vi "Waveform 64-128 channels LP pt by pt Prefilter 2.vi"(6 "order":i32=2, 8 "fl":dbl, 10 "fs":dbl, 11 "Array in":waveform(dbl)[](array[waveform])) -> (3 "Array out":waveform(dbl)[](array[waveform]))   [LabVIEW 2013]
uses:
  <vilib>/Analysis/3filter.llb/Filter Passband Type.ctl
  <vilib>/ptbypt/NI_PtbyPt.lvlib
  <vilib>/Analysis/NI_AALBase.lvlib
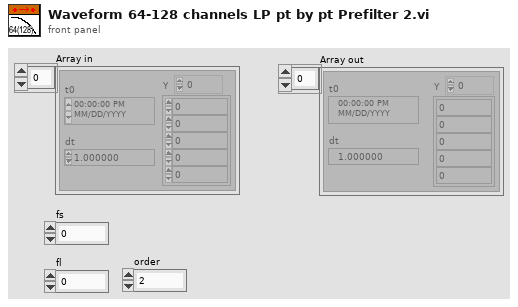
[diagram p1: front panel]
types:
  T1 = typedef "NI_AALBase.lvlib/Filter Passband Type.ctl" = enum32{"Lowpass", "Highpass", "Bandpass", "Bandstop"}
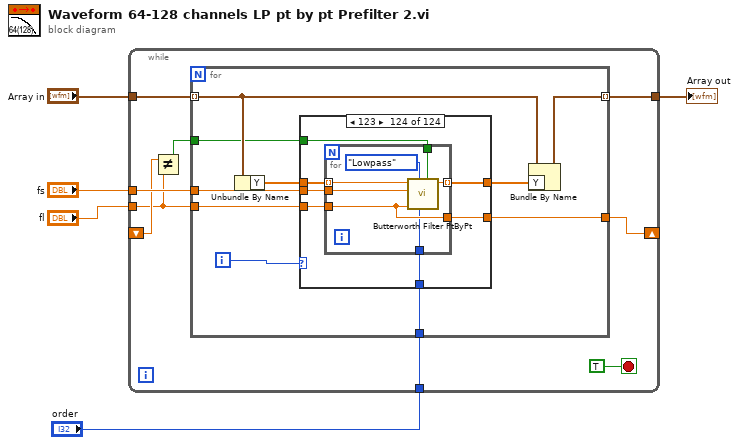
[diagram p0: block diagram]
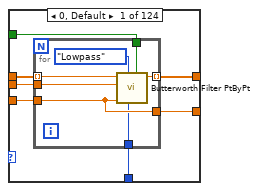
[diagram p2: hidden frame]
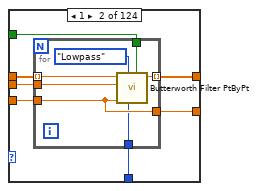
[diagram p3: hidden frame]
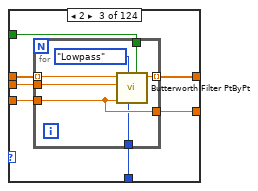
[diagram p4: hidden frame]
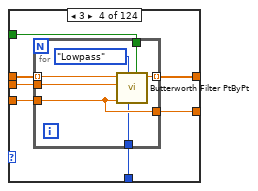
[diagram p5: hidden frame]
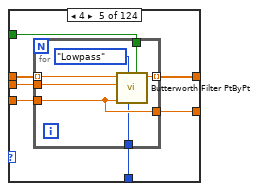
[diagram p6: hidden frame]
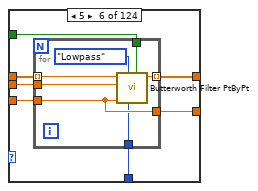
[diagram p7: hidden frame]
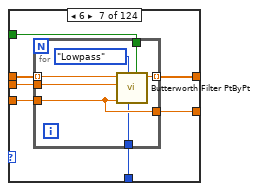
[diagram p8: hidden frame]
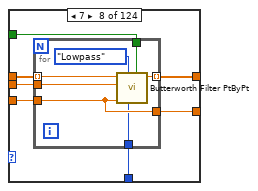
[diagram p9: hidden frame]
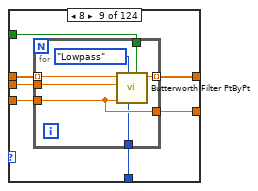
[diagram p10: hidden frame]
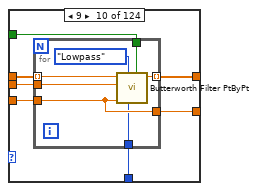
[diagram p11: hidden frame]
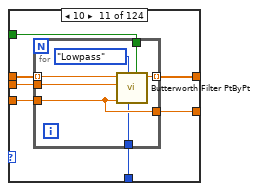
[diagram p12: hidden frame]
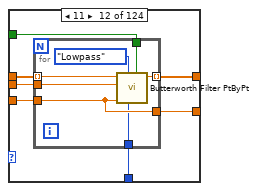
[diagram p13: hidden frame]
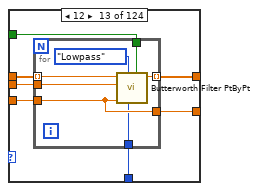
[diagram p14: hidden frame]
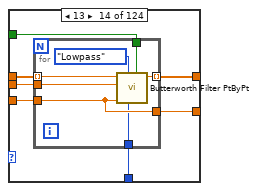
[diagram p15: hidden frame]
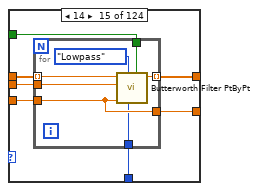
[diagram p16: hidden frame]
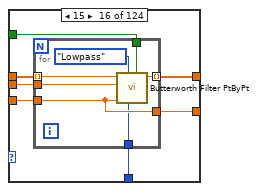
[diagram p17: hidden frame]
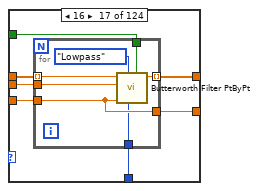
[diagram p18: hidden frame]
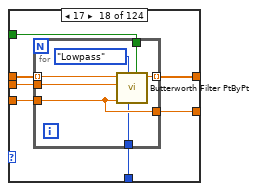
[diagram p19: hidden frame]
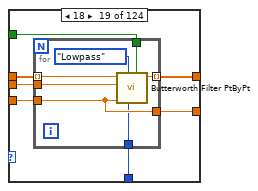
[diagram p20: hidden frame]
diagram:
  n1 = while {
    tunnel: "Array in" -> [w14]
    tunnel: [w13] -> w4
    tunnel: "fs" -> [w10]
    tunnel: "fl" -> [w7]
    shift-right: [w11] -> _
    shift-left: _ -> [w9]
    tunnel: "order" -> [w8]
    stop <- TRUE stop-if-true
    n2 = Not Equal?(x=w9, y=w7) -> (x != y?=w6:bool)
    n3 = for {
      tunnel: w14 -> [w22] mode=indexing
      tunnel: w10 -> [w24]
      tunnel: [w23] -> w13 mode=indexing
      tunnel: w7 -> [w21]
      tunnel: [w20] -> w11
      tunnel: w6 -> [w19]
      tunnel: w8 -> [w18]
      i -> [w15]
      n4 = Unbundle By Name(w22) -> ("Y"=w16:dbl[])
      n5 = case shown="123" w15 {
        tunnel: w24 -> [w31 w45 w59 w73 w87 w101 w115 w129 w143 w157 w171 w185 w199 w213 w227 w241 w255 w269 w283 w297 w311 w325 w339 w353 w367 w381 w395 w409 w423 w437 w451 w465 w479 w493 w507 w521 w535 w549 w563 w577 w591 w605 w619 w633 w647 w661 w675 w689 w703 w717 w731 w745 w759 w773 w787 w801 w815 w829 w843 w857 w871 w885 w899 w913 w927 w941 w955 w969 w983 w997 w1011 w1025 w1039 w1053 w1067 w1081 w1095 w1109 w1123 w1137 w1151 w1165 w1179 w1193 w1207 w1221 w1235 w1249 w1263 w1277 w1291 w1305 w1319 w1333 w1347 w1361 w1375 w1389 w1403 w1417 w1431 w1445 w1459 w1473 w1487 w1501 w1515 w1529 w1543 w1557 w1571 w1585 w1599 w1613 w1627 w1641 w1655 w1669 w1683 w1697 w1711 w1725 w1739 w1753]
        tunnel: w21 -> [w30 w44 w58 w72 w86 w100 w114 w128 w142 w156 w170 w184 w198 w212 w226 w240 w254 w268 w282 w296 w310 w324 w338 w352 w366 w380 w394 w408 w422 w436 w450 w464 w478 w492 w506 w520 w534 w548 w562 w576 w590 w604 w618 w632 w646 w660 w674 w688 w702 w716 w730 w744 w758 w772 w786 w800 w814 w828 w842 w856 w870 w884 w898 w912 w926 w940 w954 w968 w982 w996 w1010 w1024 w1038 w1052 w1066 w1080 w1094 w1108 w1122 w1136 w1150 w1164 w1178 w1192 w1206 w1220 w1234 w1248 w1262 w1276 w1290 w1304 w1318 w1332 w1346 w1360 w1374 w1388 w1402 w1416 w1430 w1444 w1458 w1472 w1486 w1500 w1514 w1528 w1542 w1556 w1570 w1584 w1598 w1612 w1626 w1640 w1654 w1668 w1682 w1696 w1710 w1724 w1738 w1752]
        tunnel: [w29 w43 w57 w71 w85 w99 w113 w127 w141 w155 w169 w183 w197 w211 w225 w239 w253 w267 w281 w295 w309 w323 w337 w351 w365 w379 w393 w407 w421 w435 w449 w463 w477 w491 w505 w519 w533 w547 w561 w575 w589 w603 w617 w631 w645 w659 w673 w687 w701 w715 w729 w743 w757 w771 w785 w799 w813 w827 w841 w855 w869 w883 w897 w911 w925 w939 w953 w967 w981 w995 w1009 w1023 w1037 w1051 w1065 w1079 w1093 w1107 w1121 w1135 w1149 w1163 w1177 w1191 w1205 w1219 w1233 w1247 w1261 w1275 w1289 w1303 w1317 w1331 w1345 w1359 w1373 w1387 w1401 w1415 w1429 w1443 w1457 w1471 w1485 w1499 w1513 w1527 w1541 w1555 w1569 w1583 w1597 w1611 w1625 w1639 w1653 w1667 w1681 w1695 w1709 w1723 w1737 w1751] -> w20
        tunnel: w19 -> [w28 w42 w56 w70 w84 w98 w112 w126 w140 w154 w168 w182 w196 w210 w224 w238 w252 w266 w280 w294 w308 w322 w336 w350 w364 w378 w392 w406 w420 w434 w448 w462 w476 w490 w504 w518 w532 w546 w560 w574 w588 w602 w616 w630 w644 w658 w672 w686 w700 w714 w728 w742 w756 w770 w784 w798 w812 w826 w840 w854 w868 w882 w896 w910 w924 w938 w952 w966 w980 w994 w1008 w1022 w1036 w1050 w1064 w1078 w1092 w1106 w1120 w1134 w1148 w1162 w1176 w1190 w1204 w1218 w1232 w1246 w1260 w1274 w1288 w1302 w1316 w1330 w1344 w1358 w1372 w1386 w1400 w1414 w1428 w1442 w1456 w1470 w1484 w1498 w1512 w1526 w1540 w1554 w1568 w1582 w1596 w1610 w1624 w1638 w1652 w1666 w1680 w1694 w1708 w1722 w1736 w1750]
        tunnel: w18 -> [w27 w41 w55 w69 w83 w97 w111 w125 w139 w153 w167 w181 w195 w209 w223 w237 w251 w265 w279 w293 w307 w321 w335 w349 w363 w377 w391 w405 w419 w433 w447 w461 w475 w489 w503 w517 w531 w545 w559 w573 w587 w601 w615 w629 w643 w657 w671 w685 w699 w713 w727 w741 w755 w769 w783 w797 w811 w825 w839 w853 w867 w881 w895 w909 w923 w937 w951 w965 w979 w993 w1007 w1021 w1035 w1049 w1063 w1077 w1091 w1105 w1119 w1133 w1147 w1161 w1175 w1189 w1203 w1217 w1231 w1245 w1259 w1273 w1287 w1301 w1315 w1329 w1343 w1357 w1371 w1385 w1399 w1413 w1427 w1441 w1455 w1469 w1483 w1497 w1511 w1525 w1539 w1553 w1567 w1581 w1595 w1609 w1623 w1637 w1651 w1665 w1679 w1693 w1707 w1721 w1735 w1749]
        tunnel: [w26 w40 w54 w68 w82 w96 w110 w124 w138 w152 w166 w180 w194 w208 w222 w236 w250 w264 w278 w292 w306 w320 w334 w348 w362 w376 w390 w404 w418 w432 w446 w460 w474 w488 w502 w516 w530 w544 w558 w572 w586 w600 w614 w628 w642 w656 w670 w684 w698 w712 w726 w740 w754 w768 w782 w796 w810 w824 w838 w852 w866 w880 w894 w908 w922 w936 w950 w964 w978 w992 w1006 w1020 w1034 w1048 w1062 w1076 w1090 w1104 w1118 w1132 w1146 w1160 w1174 w1188 w1202 w1216 w1230 w1244 w1258 w1272 w1286 w1300 w1314 w1328 w1342 w1356 w1370 w1384 w1398 w1412 w1426 w1440 w1454 w1468 w1482 w1496 w1510 w1524 w1538 w1552 w1566 w1580 w1594 w1608 w1622 w1636 w1650 w1664 w1678 w1692 w1706 w1720 w1734 w1748] -> w17
        tunnel: w16 -> [w25 w39 w53 w67 w81 w95 w109 w123 w137 w151 w165 w179 w193 w207 w221 w235 w249 w263 w277 w291 w305 w319 w333 w347 w361 w375 w389 w403 w417 w431 w445 w459 w473 w487 w501 w515 w529 w543 w557 w571 w585 w599 w613 w627 w641 w655 w669 w683 w697 w711 w725 w739 w753 w767 w781 w795 w809 w823 w837 w851 w865 w879 w893 w907 w921 w935 w949 w963 w977 w991 w1005 w1019 w1033 w1047 w1061 w1075 w1089 w1103 w1117 w1131 w1145 w1159 w1173 w1187 w1201 w1215 w1229 w1243 w1257 w1271 w1285 w1299 w1313 w1327 w1341 w1355 w1369 w1383 w1397 w1411 w1425 w1439 w1453 w1467 w1481 w1495 w1509 w1523 w1537 w1551 w1565 w1579 w1593 w1607 w1621 w1635 w1649 w1663 w1677 w1691 w1705 w1719 w1733 w1747]
        frame 0, Default {
          n6 = for {
            tunnel: w25 -> [w38] mode=indexing
            tunnel: w30 -> [w35]
            tunnel: w31 -> [w37]
            tunnel: [w36] -> w26 mode=indexing
            tunnel: [w35] -> w29
            tunnel: w28 -> [w33]
            tunnel: w27 -> [w32]
            n7 = call <vilib>:"Butterworth Filter PtByPt.vi"("initialize"=w33, "order"=w32, "filter type"=Filter_Passband_Type."Lowpass", "low cutoff freq: fl"=w35, "sampling freq: fs"=w37, "x"=w38) -> ("Filtered x"=w36:dbl)  [unwired: 3 in, 1 out]
          }
        }
        frame 1 {
          n8 = for {
            tunnel: w39 -> [w52] mode=indexing
            tunnel: w44 -> [w49]
            tunnel: w45 -> [w51]
            tunnel: [w50] -> w40 mode=indexing
            tunnel: [w49] -> w43
            tunnel: w42 -> [w47]
            tunnel: w41 -> [w46]
            n9 = call <vilib>:"Butterworth Filter PtByPt.vi"("initialize"=w47, "order"=w46, "filter type"=Filter_Passband_Type."Lowpass", "low cutoff freq: fl"=w49, "sampling freq: fs"=w51, "x"=w52) -> ("Filtered x"=w50:dbl)  [unwired: 3 in, 1 out]
          }
        }
        frame 2 {
          n10 = for {
            tunnel: w53 -> [w66] mode=indexing
            tunnel: w58 -> [w63]
            tunnel: w59 -> [w65]
            tunnel: [w64] -> w54 mode=indexing
            tunnel: [w63] -> w57
            tunnel: w56 -> [w61]
            tunnel: w55 -> [w60]
            n11 = call <vilib>:"Butterworth Filter PtByPt.vi"("initialize"=w61, "order"=w60, "filter type"=Filter_Passband_Type."Lowpass", "low cutoff freq: fl"=w63, "sampling freq: fs"=w65, "x"=w66) -> ("Filtered x"=w64:dbl)  [unwired: 3 in, 1 out]
          }
        }
        frame 3 {
          n12 = for {
            tunnel: w67 -> [w80] mode=indexing
            tunnel: w72 -> [w77]
            tunnel: w73 -> [w79]
            tunnel: [w78] -> w68 mode=indexing
            tunnel: [w77] -> w71
            tunnel: w70 -> [w75]
            tunnel: w69 -> [w74]
            n13 = call <vilib>:"Butterworth Filter PtByPt.vi"("initialize"=w75, "order"=w74, "filter type"=Filter_Passband_Type."Lowpass", "low cutoff freq: fl"=w77, "sampling freq: fs"=w79, "x"=w80) -> ("Filtered x"=w78:dbl)  [unwired: 3 in, 1 out]
          }
        }
        frame 4 {
          n14 = for {
            tunnel: w81 -> [w94] mode=indexing
            tunnel: w86 -> [w91]
            tunnel: w87 -> [w93]
            tunnel: [w92] -> w82 mode=indexing
            tunnel: [w91] -> w85
            tunnel: w84 -> [w89]
            tunnel: w83 -> [w88]
            n15 = call <vilib>:"Butterworth Filter PtByPt.vi"("initialize"=w89, "order"=w88, "filter type"=Filter_Passband_Type."Lowpass", "low cutoff freq: fl"=w91, "sampling freq: fs"=w93, "x"=w94) -> ("Filtered x"=w92:dbl)  [unwired: 3 in, 1 out]
          }
        }
        frame 5 {
          n16 = for {
            tunnel: w95 -> [w108] mode=indexing
            tunnel: w100 -> [w105]
            tunnel: w101 -> [w107]
            tunnel: [w106] -> w96 mode=indexing
            tunnel: [w105] -> w99
            tunnel: w98 -> [w103]
            tunnel: w97 -> [w102]
            n17 = call <vilib>:"Butterworth Filter PtByPt.vi"("initialize"=w103, "order"=w102, "filter type"=Filter_Passband_Type."Lowpass", "low cutoff freq: fl"=w105, "sampling freq: fs"=w107, "x"=w108) -> ("Filtered x"=w106:dbl)  [unwired: 3 in, 1 out]
          }
        }
        frame 6 {
          n18 = for {
            tunnel: w109 -> [w122] mode=indexing
            tunnel: w114 -> [w119]
            tunnel: w115 -> [w121]
            tunnel: [w120] -> w110 mode=indexing
            tunnel: [w119] -> w113
            tunnel: w112 -> [w117]
            tunnel: w111 -> [w116]
            n19 = call <vilib>:"Butterworth Filter PtByPt.vi"("initialize"=w117, "order"=w116, "filter type"=Filter_Passband_Type."Lowpass", "low cutoff freq: fl"=w119, "sampling freq: fs"=w121, "x"=w122) -> ("Filtered x"=w120:dbl)  [unwired: 3 in, 1 out]
          }
        }
        frame 7 {
          n20 = for {
            tunnel: w123 -> [w136] mode=indexing
            tunnel: w128 -> [w133]
            tunnel: w129 -> [w135]
            tunnel: [w134] -> w124 mode=indexing
            tunnel: [w133] -> w127
            tunnel: w126 -> [w131]
            tunnel: w125 -> [w130]
            n21 = call <vilib>:"Butterworth Filter PtByPt.vi"("initialize"=w131, "order"=w130, "filter type"=Filter_Passband_Type."Lowpass", "low cutoff freq: fl"=w133, "sampling freq: fs"=w135, "x"=w136) -> ("Filtered x"=w134:dbl)  [unwired: 3 in, 1 out]
          }
        }
        frame 8 {
          n22 = for {
            tunnel: w137 -> [w150] mode=indexing
            tunnel: w142 -> [w147]
            tunnel: w143 -> [w149]
            tunnel: [w148] -> w138 mode=indexing
            tunnel: [w147] -> w141
            tunnel: w140 -> [w145]
            tunnel: w139 -> [w144]
            n23 = call <vilib>:"Butterworth Filter PtByPt.vi"("initialize"=w145, "order"=w144, "filter type"=Filter_Passband_Type."Lowpass", "low cutoff freq: fl"=w147, "sampling freq: fs"=w149, "x"=w150) -> ("Filtered x"=w148:dbl)  [unwired: 3 in, 1 out]
          }
        }
        frame 9 {
          n24 = for {
            tunnel: w151 -> [w164] mode=indexing
            tunnel: w156 -> [w161]
            tunnel: w157 -> [w163]
            tunnel: [w162] -> w152 mode=indexing
            tunnel: [w161] -> w155
            tunnel: w154 -> [w159]
            tunnel: w153 -> [w158]
            n25 = call <vilib>:"Butterworth Filter PtByPt.vi"("initialize"=w159, "order"=w158, "filter type"=Filter_Passband_Type."Lowpass", "low cutoff freq: fl"=w161, "sampling freq: fs"=w163, "x"=w164) -> ("Filtered x"=w162:dbl)  [unwired: 3 in, 1 out]
          }
        }
        frame 10 {
          n26 = for {
            tunnel: w165 -> [w178] mode=indexing
            tunnel: w170 -> [w175]
            tunnel: w171 -> [w177]
            tunnel: [w176] -> w166 mode=indexing
            tunnel: [w175] -> w169
            tunnel: w168 -> [w173]
            tunnel: w167 -> [w172]
            n27 = call <vilib>:"Butterworth Filter PtByPt.vi"("initialize"=w173, "order"=w172, "filter type"=Filter_Passband_Type."Lowpass", "low cutoff freq: fl"=w175, "sampling freq: fs"=w177, "x"=w178) -> ("Filtered x"=w176:dbl)  [unwired: 3 in, 1 out]
          }
        }
        frame 11 {
          n28 = for {
            tunnel: w179 -> [w192] mode=indexing
            tunnel: w184 -> [w189]
            tunnel: w185 -> [w191]
            tunnel: [w190] -> w180 mode=indexing
            tunnel: [w189] -> w183
            tunnel: w182 -> [w187]
            tunnel: w181 -> [w186]
            n29 = call <vilib>:"Butterworth Filter PtByPt.vi"("initialize"=w187, "order"=w186, "filter type"=Filter_Passband_Type."Lowpass", "low cutoff freq: fl"=w189, "sampling freq: fs"=w191, "x"=w192) -> ("Filtered x"=w190:dbl)  [unwired: 3 in, 1 out]
          }
        }
        frame 12 {
          n30 = for {
            tunnel: w193 -> [w206] mode=indexing
            tunnel: w198 -> [w203]
            tunnel: w199 -> [w205]
            tunnel: [w204] -> w194 mode=indexing
            tunnel: [w203] -> w197
            tunnel: w196 -> [w201]
            tunnel: w195 -> [w200]
            n31 = call <vilib>:"Butterworth Filter PtByPt.vi"("initialize"=w201, "order"=w200, "filter type"=Filter_Passband_Type."Lowpass", "low cutoff freq: fl"=w203, "sampling freq: fs"=w205, "x"=w206) -> ("Filtered x"=w204:dbl)  [unwired: 3 in, 1 out]
          }
        }
        frame 13 {
          n32 = for {
            tunnel: w207 -> [w220] mode=indexing
            tunnel: w212 -> [w217]
            tunnel: w213 -> [w219]
            tunnel: [w218] -> w208 mode=indexing
            tunnel: [w217] -> w211
            tunnel: w210 -> [w215]
            tunnel: w209 -> [w214]
            n33 = call <vilib>:"Butterworth Filter PtByPt.vi"("initialize"=w215, "order"=w214, "filter type"=Filter_Passband_Type."Lowpass", "low cutoff freq: fl"=w217, "sampling freq: fs"=w219, "x"=w220) -> ("Filtered x"=w218:dbl)  [unwired: 3 in, 1 out]
          }
        }
        frame 14 {
          n34 = for {
            tunnel: w221 -> [w234] mode=indexing
            tunnel: w226 -> [w231]
            tunnel: w227 -> [w233]
            tunnel: [w232] -> w222 mode=indexing
            tunnel: [w231] -> w225
            tunnel: w224 -> [w229]
            tunnel: w223 -> [w228]
            n35 = call <vilib>:"Butterworth Filter PtByPt.vi"("initialize"=w229, "order"=w228, "filter type"=Filter_Passband_Type."Lowpass", "low cutoff freq: fl"=w231, "sampling freq: fs"=w233, "x"=w234) -> ("Filtered x"=w232:dbl)  [unwired: 3 in, 1 out]
          }
        }
        frame 15 {
          n36 = for {
            tunnel: w235 -> [w248] mode=indexing
            tunnel: w240 -> [w245]
            tunnel: w241 -> [w247]
            tunnel: [w246] -> w236 mode=indexing
            tunnel: [w245] -> w239
            tunnel: w238 -> [w243]
            tunnel: w237 -> [w242]
            n37 = call <vilib>:"Butterworth Filter PtByPt.vi"("initialize"=w243, "order"=w242, "filter type"=Filter_Passband_Type."Lowpass", "low cutoff freq: fl"=w245, "sampling freq: fs"=w247, "x"=w248) -> ("Filtered x"=w246:dbl)  [unwired: 3 in, 1 out]
          }
        }
        frame 16 {
          n38 = for {
            tunnel: w249 -> [w262] mode=indexing
            tunnel: w254 -> [w259]
            tunnel: w255 -> [w261]
            tunnel: [w260] -> w250 mode=indexing
            tunnel: [w259] -> w253
            tunnel: w252 -> [w257]
            tunnel: w251 -> [w256]
            n39 = call <vilib>:"Butterworth Filter PtByPt.vi"("initialize"=w257, "order"=w256, "filter type"=Filter_Passband_Type."Lowpass", "low cutoff freq: fl"=w259, "sampling freq: fs"=w261, "x"=w262) -> ("Filtered x"=w260:dbl)  [unwired: 3 in, 1 out]
          }
        }
        frame 17 {
          n40 = for {
            tunnel: w263 -> [w276] mode=indexing
            tunnel: w268 -> [w273]
            tunnel: w269 -> [w275]
            tunnel: [w274] -> w264 mode=indexing
            tunnel: [w273] -> w267
            tunnel: w266 -> [w271]
            tunnel: w265 -> [w270]
            n41 = call <vilib>:"Butterworth Filter PtByPt.vi"("initialize"=w271, "order"=w270, "filter type"=Filter_Passband_Type."Lowpass", "low cutoff freq: fl"=w273, "sampling freq: fs"=w275, "x"=w276) -> ("Filtered x"=w274:dbl)  [unwired: 3 in, 1 out]
          }
        }
        frame 18 {
          n42 = for {
            tunnel: w277 -> [w290] mode=indexing
            tunnel: w282 -> [w287]
            tunnel: w283 -> [w289]
            tunnel: [w288] -> w278 mode=indexing
            tunnel: [w287] -> w281
            tunnel: w280 -> [w285]
            tunnel: w279 -> [w284]
            n43 = call <vilib>:"Butterworth Filter PtByPt.vi"("initialize"=w285, "order"=w284, "filter type"=Filter_Passband_Type."Lowpass", "low cutoff freq: fl"=w287, "sampling freq: fs"=w289, "x"=w290) -> ("Filtered x"=w288:dbl)  [unwired: 3 in, 1 out]
          }
        }
        frame 19 {
          n44 = for {
            tunnel: w291 -> [w304] mode=indexing
            tunnel: w296 -> [w301]
            tunnel: w297 -> [w303]
            tunnel: [w302] -> w292 mode=indexing
            tunnel: [w301] -> w295
            tunnel: w294 -> [w299]
            tunnel: w293 -> [w298]
            n45 = call <vilib>:"Butterworth Filter PtByPt.vi"("initialize"=w299, "order"=w298, "filter type"=Filter_Passband_Type."Lowpass", "low cutoff freq: fl"=w301, "sampling freq: fs"=w303, "x"=w304) -> ("Filtered x"=w302:dbl)  [unwired: 3 in, 1 out]
          }
        }
        frame 20 {
          n46 = for {
            tunnel: w305 -> [w318] mode=indexing
            tunnel: w310 -> [w315]
            tunnel: w311 -> [w317]
            tunnel: [w316] -> w306 mode=indexing
            tunnel: [w315] -> w309
            tunnel: w308 -> [w313]
            tunnel: w307 -> [w312]
            n47 = call <vilib>:"Butterworth Filter PtByPt.vi"("initialize"=w313, "order"=w312, "filter type"=Filter_Passband_Type."Lowpass", "low cutoff freq: fl"=w315, "sampling freq: fs"=w317, "x"=w318) -> ("Filtered x"=w316:dbl)  [unwired: 3 in, 1 out]
          }
        }
        frame 21 {
          n48 = for {
            tunnel: w319 -> [w332] mode=indexing
            tunnel: w324 -> [w329]
            tunnel: w325 -> [w331]
            tunnel: [w330] -> w320 mode=indexing
            tunnel: [w329] -> w323
            tunnel: w322 -> [w327]
            tunnel: w321 -> [w326]
            n49 = call <vilib>:"Butterworth Filter PtByPt.vi"("initialize"=w327, "order"=w326, "filter type"=Filter_Passband_Type."Lowpass", "low cutoff freq: fl"=w329, "sampling freq: fs"=w331, "x"=w332) -> ("Filtered x"=w330:dbl)  [unwired: 3 in, 1 out]
          }
        }
        frame 22 {
          n50 = for {
            tunnel: w333 -> [w346] mode=indexing
            tunnel: w338 -> [w343]
            tunnel: w339 -> [w345]
            tunnel: [w344] -> w334 mode=indexing
            tunnel: [w343] -> w337
            tunnel: w336 -> [w341]
            tunnel: w335 -> [w340]
            n51 = call <vilib>:"Butterworth Filter PtByPt.vi"("initialize"=w341, "order"=w340, "filter type"=Filter_Passband_Type."Lowpass", "low cutoff freq: fl"=w343, "sampling freq: fs"=w345, "x"=w346) -> ("Filtered x"=w344:dbl)  [unwired: 3 in, 1 out]
          }
        }
        frame 23 {
          n52 = for {
            tunnel: w347 -> [w360] mode=indexing
            tunnel: w352 -> [w357]
            tunnel: w353 -> [w359]
            tunnel: [w358] -> w348 mode=indexing
            tunnel: [w357] -> w351
            tunnel: w350 -> [w355]
            tunnel: w349 -> [w354]
            n53 = call <vilib>:"Butterworth Filter PtByPt.vi"("initialize"=w355, "order"=w354, "filter type"=Filter_Passband_Type."Lowpass", "low cutoff freq: fl"=w357, "sampling freq: fs"=w359, "x"=w360) -> ("Filtered x"=w358:dbl)  [unwired: 3 in, 1 out]
          }
        }
        frame 24 {
          n54 = for {
            tunnel: w361 -> [w374] mode=indexing
            tunnel: w366 -> [w371]
            tunnel: w367 -> [w373]
            tunnel: [w372] -> w362 mode=indexing
            tunnel: [w371] -> w365
            tunnel: w364 -> [w369]
            tunnel: w363 -> [w368]
            n55 = call <vilib>:"Butterworth Filter PtByPt.vi"("initialize"=w369, "order"=w368, "filter type"=Filter_Passband_Type."Lowpass", "low cutoff freq: fl"=w371, "sampling freq: fs"=w373, "x"=w374) -> ("Filtered x"=w372:dbl)  [unwired: 3 in, 1 out]
          }
        }
        frame 25 {
          n56 = for {
            tunnel: w375 -> [w388] mode=indexing
            tunnel: w380 -> [w385]
            tunnel: w381 -> [w387]
            tunnel: [w386] -> w376 mode=indexing
            tunnel: [w385] -> w379
            tunnel: w378 -> [w383]
            tunnel: w377 -> [w382]
            n57 = call <vilib>:"Butterworth Filter PtByPt.vi"("initialize"=w383, "order"=w382, "filter type"=Filter_Passband_Type."Lowpass", "low cutoff freq: fl"=w385, "sampling freq: fs"=w387, "x"=w388) -> ("Filtered x"=w386:dbl)  [unwired: 3 in, 1 out]
          }
        }
        frame 26 {
          n58 = for {
            tunnel: w389 -> [w402] mode=indexing
            tunnel: w394 -> [w399]
            tunnel: w395 -> [w401]
            tunnel: [w400] -> w390 mode=indexing
            tunnel: [w399] -> w393
            tunnel: w392 -> [w397]
            tunnel: w391 -> [w396]
            n59 = call <vilib>:"Butterworth Filter PtByPt.vi"("initialize"=w397, "order"=w396, "filter type"=Filter_Passband_Type."Lowpass", "low cutoff freq: fl"=w399, "sampling freq: fs"=w401, "x"=w402) -> ("Filtered x"=w400:dbl)  [unwired: 3 in, 1 out]
          }
        }
        frame 27 {
          n60 = for {
            tunnel: w403 -> [w416] mode=indexing
            tunnel: w408 -> [w413]
            tunnel: w409 -> [w415]
            tunnel: [w414] -> w404 mode=indexing
            tunnel: [w413] -> w407
            tunnel: w406 -> [w411]
            tunnel: w405 -> [w410]
            n61 = call <vilib>:"Butterworth Filter PtByPt.vi"("initialize"=w411, "order"=w410, "filter type"=Filter_Passband_Type."Lowpass", "low cutoff freq: fl"=w413, "sampling freq: fs"=w415, "x"=w416) -> ("Filtered x"=w414:dbl)  [unwired: 3 in, 1 out]
          }
        }
        frame 28 {
          n62 = for {
            tunnel: w417 -> [w430] mode=indexing
            tunnel: w422 -> [w427]
            tunnel: w423 -> [w429]
            tunnel: [w428] -> w418 mode=indexing
            tunnel: [w427] -> w421
            tunnel: w420 -> [w425]
            tunnel: w419 -> [w424]
            n63 = call <vilib>:"Butterworth Filter PtByPt.vi"("initialize"=w425, "order"=w424, "filter type"=Filter_Passband_Type."Lowpass", "low cutoff freq: fl"=w427, "sampling freq: fs"=w429, "x"=w430) -> ("Filtered x"=w428:dbl)  [unwired: 3 in, 1 out]
          }
        }
        frame 29 {
          n64 = for {
            tunnel: w431 -> [w444] mode=indexing
            tunnel: w436 -> [w441]
            tunnel: w437 -> [w443]
            tunnel: [w442] -> w432 mode=indexing
            tunnel: [w441] -> w435
            tunnel: w434 -> [w439]
            tunnel: w433 -> [w438]
            n65 = call <vilib>:"Butterworth Filter PtByPt.vi"("initialize"=w439, "order"=w438, "filter type"=Filter_Passband_Type."Lowpass", "low cutoff freq: fl"=w441, "sampling freq: fs"=w443, "x"=w444) -> ("Filtered x"=w442:dbl)  [unwired: 3 in, 1 out]
          }
        }
        frame 30 {
          n66 = for {
            tunnel: w445 -> [w458] mode=indexing
            tunnel: w450 -> [w455]
            tunnel: w451 -> [w457]
            tunnel: [w456] -> w446 mode=indexing
            tunnel: [w455] -> w449
            tunnel: w448 -> [w453]
            tunnel: w447 -> [w452]
            n67 = call <vilib>:"Butterworth Filter PtByPt.vi"("initialize"=w453, "order"=w452, "filter type"=Filter_Passband_Type."Lowpass", "low cutoff freq: fl"=w455, "sampling freq: fs"=w457, "x"=w458) -> ("Filtered x"=w456:dbl)  [unwired: 3 in, 1 out]
          }
        }
        frame 31 {
          n68 = for {
            tunnel: w459 -> [w472] mode=indexing
            tunnel: w464 -> [w469]
            tunnel: w465 -> [w471]
            tunnel: [w470] -> w460 mode=indexing
            tunnel: [w469] -> w463
            tunnel: w462 -> [w467]
            tunnel: w461 -> [w466]
            n69 = call <vilib>:"Butterworth Filter PtByPt.vi"("initialize"=w467, "order"=w466, "filter type"=Filter_Passband_Type."Lowpass", "low cutoff freq: fl"=w469, "sampling freq: fs"=w471, "x"=w472) -> ("Filtered x"=w470:dbl)  [unwired: 3 in, 1 out]
          }
        }
        frame 32 {
          n70 = for {
            tunnel: w473 -> [w486] mode=indexing
            tunnel: w478 -> [w483]
            tunnel: w479 -> [w485]
            tunnel: [w484] -> w474 mode=indexing
            tunnel: [w483] -> w477
            tunnel: w476 -> [w481]
            tunnel: w475 -> [w480]
            n71 = call <vilib>:"Butterworth Filter PtByPt.vi"("initialize"=w481, "order"=w480, "filter type"=Filter_Passband_Type."Lowpass", "low cutoff freq: fl"=w483, "sampling freq: fs"=w485, "x"=w486) -> ("Filtered x"=w484:dbl)  [unwired: 3 in, 1 out]
          }
        }
        frame 33 {
          n72 = for {
            tunnel: w487 -> [w500] mode=indexing
            tunnel: w492 -> [w497]
            tunnel: w493 -> [w499]
            tunnel: [w498] -> w488 mode=indexing
            tunnel: [w497] -> w491
            tunnel: w490 -> [w495]
            tunnel: w489 -> [w494]
            n73 = call <vilib>:"Butterworth Filter PtByPt.vi"("initialize"=w495, "order"=w494, "filter type"=Filter_Passband_Type."Lowpass", "low cutoff freq: fl"=w497, "sampling freq: fs"=w499, "x"=w500) -> ("Filtered x"=w498:dbl)  [unwired: 3 in, 1 out]
          }
        }
        frame 34 {
          n74 = for {
            tunnel: w501 -> [w514] mode=indexing
            tunnel: w506 -> [w511]
            tunnel: w507 -> [w513]
            tunnel: [w512] -> w502 mode=indexing
            tunnel: [w511] -> w505
            tunnel: w504 -> [w509]
            tunnel: w503 -> [w508]
            n75 = call <vilib>:"Butterworth Filter PtByPt.vi"("initialize"=w509, "order"=w508, "filter type"=Filter_Passband_Type."Lowpass", "low cutoff freq: fl"=w511, "sampling freq: fs"=w513, "x"=w514) -> ("Filtered x"=w512:dbl)  [unwired: 3 in, 1 out]
          }
        }
        frame 35 {
          n76 = for {
            tunnel: w515 -> [w528] mode=indexing
            tunnel: w520 -> [w525]
            tunnel: w521 -> [w527]
            tunnel: [w526] -> w516 mode=indexing
            tunnel: [w525] -> w519
            tunnel: w518 -> [w523]
            tunnel: w517 -> [w522]
            n77 = call <vilib>:"Butterworth Filter PtByPt.vi"("initialize"=w523, "order"=w522, "filter type"=Filter_Passband_Type."Lowpass", "low cutoff freq: fl"=w525, "sampling freq: fs"=w527, "x"=w528) -> ("Filtered x"=w526:dbl)  [unwired: 3 in, 1 out]
          }
        }
        frame 36 {
          n78 = for {
            tunnel: w529 -> [w542] mode=indexing
            tunnel: w534 -> [w539]
            tunnel: w535 -> [w541]
            tunnel: [w540] -> w530 mode=indexing
            tunnel: [w539] -> w533
            tunnel: w532 -> [w537]
            tunnel: w531 -> [w536]
            n79 = call <vilib>:"Butterworth Filter PtByPt.vi"("initialize"=w537, "order"=w536, "filter type"=Filter_Passband_Type."Lowpass", "low cutoff freq: fl"=w539, "sampling freq: fs"=w541, "x"=w542) -> ("Filtered x"=w540:dbl)  [unwired: 3 in, 1 out]
          }
        }
        frame 37 {
          n80 = for {
            tunnel: w543 -> [w556] mode=indexing
            tunnel: w548 -> [w553]
            tunnel: w549 -> [w555]
            tunnel: [w554] -> w544 mode=indexing
            tunnel: [w553] -> w547
            tunnel: w546 -> [w551]
            tunnel: w545 -> [w550]
            n81 = call <vilib>:"Butterworth Filter PtByPt.vi"("initialize"=w551, "order"=w550, "filter type"=Filter_Passband_Type."Lowpass", "low cutoff freq: fl"=w553, "sampling freq: fs"=w555, "x"=w556) -> ("Filtered x"=w554:dbl)  [unwired: 3 in, 1 out]
          }
        }
        frame 38 {
          n82 = for {
            tunnel: w557 -> [w570] mode=indexing
            tunnel: w562 -> [w567]
            tunnel: w563 -> [w569]
            tunnel: [w568] -> w558 mode=indexing
            tunnel: [w567] -> w561
            tunnel: w560 -> [w565]
            tunnel: w559 -> [w564]
            n83 = call <vilib>:"Butterworth Filter PtByPt.vi"("initialize"=w565, "order"=w564, "filter type"=Filter_Passband_Type."Lowpass", "low cutoff freq: fl"=w567, "sampling freq: fs"=w569, "x"=w570) -> ("Filtered x"=w568:dbl)  [unwired: 3 in, 1 out]
          }
        }
        frame 39 {
          n84 = for {
            tunnel: w571 -> [w584] mode=indexing
            tunnel: w576 -> [w581]
            tunnel: w577 -> [w583]
            tunnel: [w582] -> w572 mode=indexing
            tunnel: [w581] -> w575
            tunnel: w574 -> [w579]
            tunnel: w573 -> [w578]
            n85 = call <vilib>:"Butterworth Filter PtByPt.vi"("initialize"=w579, "order"=w578, "filter type"=Filter_Passband_Type."Lowpass", "low cutoff freq: fl"=w581, "sampling freq: fs"=w583, "x"=w584) -> ("Filtered x"=w582:dbl)  [unwired: 3 in, 1 out]
          }
        }
        frame 40 {
          n86 = for {
            tunnel: w585 -> [w598] mode=indexing
            tunnel: w590 -> [w595]
            tunnel: w591 -> [w597]
            tunnel: [w596] -> w586 mode=indexing
            tunnel: [w595] -> w589
            tunnel: w588 -> [w593]
            tunnel: w587 -> [w592]
            n87 = call <vilib>:"Butterworth Filter PtByPt.vi"("initialize"=w593, "order"=w592, "filter type"=Filter_Passband_Type."Lowpass", "low cutoff freq: fl"=w595, "sampling freq: fs"=w597, "x"=w598) -> ("Filtered x"=w596:dbl)  [unwired: 3 in, 1 out]
          }
        }
        frame 41 {
          n88 = for {
            tunnel: w599 -> [w612] mode=indexing
            tunnel: w604 -> [w609]
            tunnel: w605 -> [w611]
            tunnel: [w610] -> w600 mode=indexing
            tunnel: [w609] -> w603
            tunnel: w602 -> [w607]
            tunnel: w601 -> [w606]
            n89 = call <vilib>:"Butterworth Filter PtByPt.vi"("initialize"=w607, "order"=w606, "filter type"=Filter_Passband_Type."Lowpass", "low cutoff freq: fl"=w609, "sampling freq: fs"=w611, "x"=w612) -> ("Filtered x"=w610:dbl)  [unwired: 3 in, 1 out]
          }
        }
        frame 42 {
          n90 = for {
            tunnel: w613 -> [w626] mode=indexing
            tunnel: w618 -> [w623]
            tunnel: w619 -> [w625]
            tunnel: [w624] -> w614 mode=indexing
            tunnel: [w623] -> w617
            tunnel: w616 -> [w621]
            tunnel: w615 -> [w620]
            n91 = call <vilib>:"Butterworth Filter PtByPt.vi"("initialize"=w621, "order"=w620, "filter type"=Filter_Passband_Type."Lowpass", "low cutoff freq: fl"=w623, "sampling freq: fs"=w625, "x"=w626) -> ("Filtered x"=w624:dbl)  [unwired: 3 in, 1 out]
          }
        }
        frame 43 {
          n92 = for {
            tunnel: w627 -> [w640] mode=indexing
            tunnel: w632 -> [w637]
            tunnel: w633 -> [w639]
            tunnel: [w638] -> w628 mode=indexing
            tunnel: [w637] -> w631
            tunnel: w630 -> [w635]
            tunnel: w629 -> [w634]
            n93 = call <vilib>:"Butterworth Filter PtByPt.vi"("initialize"=w635, "order"=w634, "filter type"=Filter_Passband_Type."Lowpass", "low cutoff freq: fl"=w637, "sampling freq: fs"=w639, "x"=w640) -> ("Filtered x"=w638:dbl)  [unwired: 3 in, 1 out]
          }
        }
        frame 44 {
          n94 = for {
            tunnel: w641 -> [w654] mode=indexing
            tunnel: w646 -> [w651]
            tunnel: w647 -> [w653]
            tunnel: [w652] -> w642 mode=indexing
            tunnel: [w651] -> w645
            tunnel: w644 -> [w649]
            tunnel: w643 -> [w648]
            n95 = call <vilib>:"Butterworth Filter PtByPt.vi"("initialize"=w649, "order"=w648, "filter type"=Filter_Passband_Type."Lowpass", "low cutoff freq: fl"=w651, "sampling freq: fs"=w653, "x"=w654) -> ("Filtered x"=w652:dbl)  [unwired: 3 in, 1 out]
          }
        }
        frame 45 {
          n96 = for {
            tunnel: w655 -> [w668] mode=indexing
            tunnel: w660 -> [w665]
            tunnel: w661 -> [w667]
            tunnel: [w666] -> w656 mode=indexing
            tunnel: [w665] -> w659
            tunnel: w658 -> [w663]
            tunnel: w657 -> [w662]
            n97 = call <vilib>:"Butterworth Filter PtByPt.vi"("initialize"=w663, "order"=w662, "filter type"=Filter_Passband_Type."Lowpass", "low cutoff freq: fl"=w665, "sampling freq: fs"=w667, "x"=w668) -> ("Filtered x"=w666:dbl)  [unwired: 3 in, 1 out]
          }
        }
        frame 46 {
          n98 = for {
            tunnel: w669 -> [w682] mode=indexing
            tunnel: w674 -> [w679]
            tunnel: w675 -> [w681]
            tunnel: [w680] -> w670 mode=indexing
            tunnel: [w679] -> w673
            tunnel: w672 -> [w677]
            tunnel: w671 -> [w676]
            n99 = call <vilib>:"Butterworth Filter PtByPt.vi"("initialize"=w677, "order"=w676, "filter type"=Filter_Passband_Type."Lowpass", "low cutoff freq: fl"=w679, "sampling freq: fs"=w681, "x"=w682) -> ("Filtered x"=w680:dbl)  [unwired: 3 in, 1 out]
          }
        }
        frame 47 {
          n100 = for {
            tunnel: w683 -> [w696] mode=indexing
            tunnel: w688 -> [w693]
            tunnel: w689 -> [w695]
            tunnel: [w694] -> w684 mode=indexing
            tunnel: [w693] -> w687
            tunnel: w686 -> [w691]
            tunnel: w685 -> [w690]
            n101 = call <vilib>:"Butterworth Filter PtByPt.vi"("initialize"=w691, "order"=w690, "filter type"=Filter_Passband_Type."Lowpass", "low cutoff freq: fl"=w693, "sampling freq: fs"=w695, "x"=w696) -> ("Filtered x"=w694:dbl)  [unwired: 3 in, 1 out]
          }
        }
        frame 48 {
          n102 = for {
            tunnel: w697 -> [w710] mode=indexing
            tunnel: w702 -> [w707]
            tunnel: w703 -> [w709]
            tunnel: [w708] -> w698 mode=indexing
            tunnel: [w707] -> w701
            tunnel: w700 -> [w705]
            tunnel: w699 -> [w704]
            n103 = call <vilib>:"Butterworth Filter PtByPt.vi"("initialize"=w705, "order"=w704, "filter type"=Filter_Passband_Type."Lowpass", "low cutoff freq: fl"=w707, "sampling freq: fs"=w709, "x"=w710) -> ("Filtered x"=w708:dbl)  [unwired: 3 in, 1 out]
          }
        }
        frame 49 {
          n104 = for {
            tunnel: w711 -> [w724] mode=indexing
            tunnel: w716 -> [w721]
            tunnel: w717 -> [w723]
            tunnel: [w722] -> w712 mode=indexing
            tunnel: [w721] -> w715
            tunnel: w714 -> [w719]
            tunnel: w713 -> [w718]
            n105 = call <vilib>:"Butterworth Filter PtByPt.vi"("initialize"=w719, "order"=w718, "filter type"=Filter_Passband_Type."Lowpass", "low cutoff freq: fl"=w721, "sampling freq: fs"=w723, "x"=w724) -> ("Filtered x"=w722:dbl)  [unwired: 3 in, 1 out]
          }
        }
        frame 50 {
          n106 = for {
            tunnel: w725 -> [w738] mode=indexing
            tunnel: w730 -> [w735]
            tunnel: w731 -> [w737]
            tunnel: [w736] -> w726 mode=indexing
            tunnel: [w735] -> w729
            tunnel: w728 -> [w733]
            tunnel: w727 -> [w732]
            n107 = call <vilib>:"Butterworth Filter PtByPt.vi"("initialize"=w733, "order"=w732, "filter type"=Filter_Passband_Type."Lowpass", "low cutoff freq: fl"=w735, "sampling freq: fs"=w737, "x"=w738) -> ("Filtered x"=w736:dbl)  [unwired: 3 in, 1 out]
          }
        }
        frame 51 {
          n108 = for {
            tunnel: w739 -> [w752] mode=indexing
            tunnel: w744 -> [w749]
            tunnel: w745 -> [w751]
            tunnel: [w750] -> w740 mode=indexing
            tunnel: [w749] -> w743
            tunnel: w742 -> [w747]
            tunnel: w741 -> [w746]
            n109 = call <vilib>:"Butterworth Filter PtByPt.vi"("initialize"=w747, "order"=w746, "filter type"=Filter_Passband_Type."Lowpass", "low cutoff freq: fl"=w749, "sampling freq: fs"=w751, "x"=w752) -> ("Filtered x"=w750:dbl)  [unwired: 3 in, 1 out]
          }
        }
        frame 52 {
          n110 = for {
            tunnel: w753 -> [w766] mode=indexing
            tunnel: w758 -> [w763]
            tunnel: w759 -> [w765]
            tunnel: [w764] -> w754 mode=indexing
            tunnel: [w763] -> w757
            tunnel: w756 -> [w761]
            tunnel: w755 -> [w760]
            n111 = call <vilib>:"Butterworth Filter PtByPt.vi"("initialize"=w761, "order"=w760, "filter type"=Filter_Passband_Type."Lowpass", "low cutoff freq: fl"=w763, "sampling freq: fs"=w765, "x"=w766) -> ("Filtered x"=w764:dbl)  [unwired: 3 in, 1 out]
          }
        }
        frame 53 {
          n112 = for {
            tunnel: w767 -> [w780] mode=indexing
            tunnel: w772 -> [w777]
            tunnel: w773 -> [w779]
            tunnel: [w778] -> w768 mode=indexing
            tunnel: [w777] -> w771
            tunnel: w770 -> [w775]
            tunnel: w769 -> [w774]
            n113 = call <vilib>:"Butterworth Filter PtByPt.vi"("initialize"=w775, "order"=w774, "filter type"=Filter_Passband_Type."Lowpass", "low cutoff freq: fl"=w777, "sampling freq: fs"=w779, "x"=w780) -> ("Filtered x"=w778:dbl)  [unwired: 3 in, 1 out]
          }
        }
        frame 54 {
          n114 = for {
            tunnel: w781 -> [w794] mode=indexing
            tunnel: w786 -> [w791]
            tunnel: w787 -> [w793]
            tunnel: [w792] -> w782 mode=indexing
            tunnel: [w791] -> w785
            tunnel: w784 -> [w789]
            tunnel: w783 -> [w788]
            n115 = call <vilib>:"Butterworth Filter PtByPt.vi"("initialize"=w789, "order"=w788, "filter type"=Filter_Passband_Type."Lowpass", "low cutoff freq: fl"=w791, "sampling freq: fs"=w793, "x"=w794) -> ("Filtered x"=w792:dbl)  [unwired: 3 in, 1 out]
          }
        }
        frame 55 {
          n116 = for {
            tunnel: w795 -> [w808] mode=indexing
            tunnel: w800 -> [w805]
            tunnel: w801 -> [w807]
            tunnel: [w806] -> w796 mode=indexing
            tunnel: [w805] -> w799
            tunnel: w798 -> [w803]
            tunnel: w797 -> [w802]
            n117 = call <vilib>:"Butterworth Filter PtByPt.vi"("initialize"=w803, "order"=w802, "filter type"=Filter_Passband_Type."Lowpass", "low cutoff freq: fl"=w805, "sampling freq: fs"=w807, "x"=w808) -> ("Filtered x"=w806:dbl)  [unwired: 3 in, 1 out]
          }
        }
        frame 56 {
          n118 = for {
            tunnel: w809 -> [w822] mode=indexing
            tunnel: w814 -> [w819]
            tunnel: w815 -> [w821]
            tunnel: [w820] -> w810 mode=indexing
            tunnel: [w819] -> w813
            tunnel: w812 -> [w817]
            tunnel: w811 -> [w816]
            n119 = call <vilib>:"Butterworth Filter PtByPt.vi"("initialize"=w817, "order"=w816, "filter type"=Filter_Passband_Type."Lowpass", "low cutoff freq: fl"=w819, "sampling freq: fs"=w821, "x"=w822) -> ("Filtered x"=w820:dbl)  [unwired: 3 in, 1 out]
          }
        }
        frame 57 {
          n120 = for {
            tunnel: w823 -> [w836] mode=indexing
            tunnel: w828 -> [w833]
            tunnel: w829 -> [w835]
            tunnel: [w834] -> w824 mode=indexing
            tunnel: [w833] -> w827
            tunnel: w826 -> [w831]
            tunnel: w825 -> [w830]
            n121 = call <vilib>:"Butterworth Filter PtByPt.vi"("initialize"=w831, "order"=w830, "filter type"=Filter_Passband_Type."Lowpass", "low cutoff freq: fl"=w833, "sampling freq: fs"=w835, "x"=w836) -> ("Filtered x"=w834:dbl)  [unwired: 3 in, 1 out]
          }
        }
        frame 58 {
          n122 = for {
            tunnel: w837 -> [w850] mode=indexing
            tunnel: w842 -> [w847]
            tunnel: w843 -> [w849]
            tunnel: [w848] -> w838 mode=indexing
            tunnel: [w847] -> w841
            tunnel: w840 -> [w845]
            tunnel: w839 -> [w844]
            n123 = call <vilib>:"Butterworth Filter PtByPt.vi"("initialize"=w845, "order"=w844, "filter type"=Filter_Passband_Type."Lowpass", "low cutoff freq: fl"=w847, "sampling freq: fs"=w849, "x"=w850) -> ("Filtered x"=w848:dbl)  [unwired: 3 in, 1 out]
          }
        }
        frame 59 {
          n124 = for {
            tunnel: w851 -> [w864] mode=indexing
            tunnel: w856 -> [w861]
            tunnel: w857 -> [w863]
            tunnel: [w862] -> w852 mode=indexing
            tunnel: [w861] -> w855
            tunnel: w854 -> [w859]
            tunnel: w853 -> [w858]
            n125 = call <vilib>:"Butterworth Filter PtByPt.vi"("initialize"=w859, "order"=w858, "filter type"=Filter_Passband_Type."Lowpass", "low cutoff freq: fl"=w861, "sampling freq: fs"=w863, "x"=w864) -> ("Filtered x"=w862:dbl)  [unwired: 3 in, 1 out]
          }
        }
        frame 60 {
          n126 = for {
            tunnel: w865 -> [w878] mode=indexing
            tunnel: w870 -> [w875]
            tunnel: w871 -> [w877]
            tunnel: [w876] -> w866 mode=indexing
            tunnel: [w875] -> w869
            tunnel: w868 -> [w873]
            tunnel: w867 -> [w872]
            n127 = call <vilib>:"Butterworth Filter PtByPt.vi"("initialize"=w873, "order"=w872, "filter type"=Filter_Passband_Type."Lowpass", "low cutoff freq: fl"=w875, "sampling freq: fs"=w877, "x"=w878) -> ("Filtered x"=w876:dbl)  [unwired: 3 in, 1 out]
          }
        }
        frame 61 {
          n128 = for {
            tunnel: w879 -> [w892] mode=indexing
            tunnel: w884 -> [w889]
            tunnel: w885 -> [w891]
            tunnel: [w890] -> w880 mode=indexing
            tunnel: [w889] -> w883
            tunnel: w882 -> [w887]
            tunnel: w881 -> [w886]
            n129 = call <vilib>:"Butterworth Filter PtByPt.vi"("initialize"=w887, "order"=w886, "filter type"=Filter_Passband_Type."Lowpass", "low cutoff freq: fl"=w889, "sampling freq: fs"=w891, "x"=w892) -> ("Filtered x"=w890:dbl)  [unwired: 3 in, 1 out]
          }
        }
        frame 62 {
          n130 = for {
            tunnel: w893 -> [w906] mode=indexing
            tunnel: w898 -> [w903]
            tunnel: w899 -> [w905]
            tunnel: [w904] -> w894 mode=indexing
            tunnel: [w903] -> w897
            tunnel: w896 -> [w901]
            tunnel: w895 -> [w900]
            n131 = call <vilib>:"Butterworth Filter PtByPt.vi"("initialize"=w901, "order"=w900, "filter type"=Filter_Passband_Type."Lowpass", "low cutoff freq: fl"=w903, "sampling freq: fs"=w905, "x"=w906) -> ("Filtered x"=w904:dbl)  [unwired: 3 in, 1 out]
          }
        }
        frame 63 {
          n132 = for {
            tunnel: w907 -> [w920] mode=indexing
            tunnel: w912 -> [w917]
            tunnel: w913 -> [w919]
            tunnel: [w918] -> w908 mode=indexing
            tunnel: [w917] -> w911
            tunnel: w910 -> [w915]
            tunnel: w909 -> [w914]
            n133 = call <vilib>:"Butterworth Filter PtByPt.vi"("initialize"=w915, "order"=w914, "filter type"=Filter_Passband_Type."Lowpass", "low cutoff freq: fl"=w917, "sampling freq: fs"=w919, "x"=w920) -> ("Filtered x"=w918:dbl)  [unwired: 3 in, 1 out]
          }
        }
        frame 64 {
          n134 = for {
            tunnel: w921 -> [w934] mode=indexing
            tunnel: w926 -> [w931]
            tunnel: w927 -> [w933]
            tunnel: [w932] -> w922 mode=indexing
            tunnel: [w931] -> w925
            tunnel: w924 -> [w929]
            tunnel: w923 -> [w928]
            n135 = call <vilib>:"Butterworth Filter PtByPt.vi"("initialize"=w929, "order"=w928, "filter type"=Filter_Passband_Type."Lowpass", "low cutoff freq: fl"=w931, "sampling freq: fs"=w933, "x"=w934) -> ("Filtered x"=w932:dbl)  [unwired: 3 in, 1 out]
          }
        }
        frame 65 {
          n136 = for {
            tunnel: w935 -> [w948] mode=indexing
            tunnel: w940 -> [w945]
            tunnel: w941 -> [w947]
            tunnel: [w946] -> w936 mode=indexing
            tunnel: [w945] -> w939
            tunnel: w938 -> [w943]
            tunnel: w937 -> [w942]
            n137 = call <vilib>:"Butterworth Filter PtByPt.vi"("initialize"=w943, "order"=w942, "filter type"=Filter_Passband_Type."Lowpass", "low cutoff freq: fl"=w945, "sampling freq: fs"=w947, "x"=w948) -> ("Filtered x"=w946:dbl)  [unwired: 3 in, 1 out]
          }
        }
        frame 66 {
          n138 = for {
            tunnel: w949 -> [w962] mode=indexing
            tunnel: w954 -> [w959]
            tunnel: w955 -> [w961]
            tunnel: [w960] -> w950 mode=indexing
            tunnel: [w959] -> w953
            tunnel: w952 -> [w957]
            tunnel: w951 -> [w956]
            n139 = call <vilib>:"Butterworth Filter PtByPt.vi"("initialize"=w957, "order"=w956, "filter type"=Filter_Passband_Type."Lowpass", "low cutoff freq: fl"=w959, "sampling freq: fs"=w961, "x"=w962) -> ("Filtered x"=w960:dbl)  [unwired: 3 in, 1 out]
          }
        }
        frame 67 {
          n140 = for {
            tunnel: w963 -> [w976] mode=indexing
            tunnel: w968 -> [w973]
            tunnel: w969 -> [w975]
            tunnel: [w974] -> w964 mode=indexing
            tunnel: [w973] -> w967
            tunnel: w966 -> [w971]
            tunnel: w965 -> [w970]
            n141 = call <vilib>:"Butterworth Filter PtByPt.vi"("initialize"=w971, "order"=w970, "filter type"=Filter_Passband_Type."Lowpass", "low cutoff freq: fl"=w973, "sampling freq: fs"=w975, "x"=w976) -> ("Filtered x"=w974:dbl)  [unwired: 3 in, 1 out]
          }
        }
        frame 68 {
          n142 = for {
            tunnel: w977 -> [w990] mode=indexing
            tunnel: w982 -> [w987]
            tunnel: w983 -> [w989]
            tunnel: [w988] -> w978 mode=indexing
            tunnel: [w987] -> w981
            tunnel: w980 -> [w985]
            tunnel: w979 -> [w984]
            n143 = call <vilib>:"Butterworth Filter PtByPt.vi"("initialize"=w985, "order"=w984, "filter type"=Filter_Passband_Type."Lowpass", "low cutoff freq: fl"=w987, "sampling freq: fs"=w989, "x"=w990) -> ("Filtered x"=w988:dbl)  [unwired: 3 in, 1 out]
          }
        }
        frame 69 {
          n144 = for {
            tunnel: w991 -> [w1004] mode=indexing
            tunnel: w996 -> [w1001]
            tunnel: w997 -> [w1003]
            tunnel: [w1002] -> w992 mode=indexing
            tunnel: [w1001] -> w995
            tunnel: w994 -> [w999]
            tunnel: w993 -> [w998]
            n145 = call <vilib>:"Butterworth Filter PtByPt.vi"("initialize"=w999, "order"=w998, "filter type"=Filter_Passband_Type."Lowpass", "low cutoff freq: fl"=w1001, "sampling freq: fs"=w1003, "x"=w1004) -> ("Filtered x"=w1002:dbl)  [unwired: 3 in, 1 out]
          }
        }
        frame 70 {
          n146 = for {
            tunnel: w1005 -> [w1018] mode=indexing
            tunnel: w1010 -> [w1015]
            tunnel: w1011 -> [w1017]
            tunnel: [w1016] -> w1006 mode=indexing
            tunnel: [w1015] -> w1009
            tunnel: w1008 -> [w1013]
            tunnel: w1007 -> [w1012]
            n147 = call <vilib>:"Butterworth Filter PtByPt.vi"("initialize"=w1013, "order"=w1012, "filter type"=Filter_Passband_Type."Lowpass", "low cutoff freq: fl"=w1015, "sampling freq: fs"=w1017, "x"=w1018) -> ("Filtered x"=w1016:dbl)  [unwired: 3 in, 1 out]
          }
        }
        frame 71 {
          n148 = for {
            tunnel: w1019 -> [w1032] mode=indexing
            tunnel: w1024 -> [w1029]
            tunnel: w1025 -> [w1031]
            tunnel: [w1030] -> w1020 mode=indexing
            tunnel: [w1029] -> w1023
            tunnel: w1022 -> [w1027]
            tunnel: w1021 -> [w1026]
            n149 = call <vilib>:"Butterworth Filter PtByPt.vi"("initialize"=w1027, "order"=w1026, "filter type"=Filter_Passband_Type."Lowpass", "low cutoff freq: fl"=w1029, "sampling freq: fs"=w1031, "x"=w1032) -> ("Filtered x"=w1030:dbl)  [unwired: 3 in, 1 out]
          }
        }
        frame 72 {
          n150 = for {
            tunnel: w1033 -> [w1046] mode=indexing
            tunnel: w1038 -> [w1043]
            tunnel: w1039 -> [w1045]
            tunnel: [w1044] -> w1034 mode=indexing
            tunnel: [w1043] -> w1037
            tunnel: w1036 -> [w1041]
            tunnel: w1035 -> [w1040]
            n151 = call <vilib>:"Butterworth Filter PtByPt.vi"("initialize"=w1041, "order"=w1040, "filter type"=Filter_Passband_Type."Lowpass", "low cutoff freq: fl"=w1043, "sampling freq: fs"=w1045, "x"=w1046) -> ("Filtered x"=w1044:dbl)  [unwired: 3 in, 1 out]
          }
        }
        frame 73 {
          n152 = for {
            tunnel: w1047 -> [w1060] mode=indexing
            tunnel: w1052 -> [w1057]
            tunnel: w1053 -> [w1059]
            tunnel: [w1058] -> w1048 mode=indexing
            tunnel: [w1057] -> w1051
            tunnel: w1050 -> [w1055]
            tunnel: w1049 -> [w1054]
            n153 = call <vilib>:"Butterworth Filter PtByPt.vi"("initialize"=w1055, "order"=w1054, "filter type"=Filter_Passband_Type."Lowpass", "low cutoff freq: fl"=w1057, "sampling freq: fs"=w1059, "x"=w1060) -> ("Filtered x"=w1058:dbl)  [unwired: 3 in, 1 out]
          }
        }
        frame 74 {
          n154 = for {
            tunnel: w1061 -> [w1074] mode=indexing
            tunnel: w1066 -> [w1071]
            tunnel: w1067 -> [w1073]
            tunnel: [w1072] -> w1062 mode=indexing
            tunnel: [w1071] -> w1065
            tunnel: w1064 -> [w1069]
            tunnel: w1063 -> [w1068]
            n155 = call <vilib>:"Butterworth Filter PtByPt.vi"("initialize"=w1069, "order"=w1068, "filter type"=Filter_Passband_Type."Lowpass", "low cutoff freq: fl"=w1071, "sampling freq: fs"=w1073, "x"=w1074) -> ("Filtered x"=w1072:dbl)  [unwired: 3 in, 1 out]
          }
        }
        frame 75 {
          n156 = for {
            tunnel: w1075 -> [w1088] mode=indexing
            tunnel: w1080 -> [w1085]
            tunnel: w1081 -> [w1087]
            tunnel: [w1086] -> w1076 mode=indexing
            tunnel: [w1085] -> w1079
            tunnel: w1078 -> [w1083]
            tunnel: w1077 -> [w1082]
            n157 = call <vilib>:"Butterworth Filter PtByPt.vi"("initialize"=w1083, "order"=w1082, "filter type"=Filter_Passband_Type."Lowpass", "low cutoff freq: fl"=w1085, "sampling freq: fs"=w1087, "x"=w1088) -> ("Filtered x"=w1086:dbl)  [unwired: 3 in, 1 out]
          }
        }
        frame 76 {
          n158 = for {
            tunnel: w1089 -> [w1102] mode=indexing
            tunnel: w1094 -> [w1099]
            tunnel: w1095 -> [w1101]
            tunnel: [w1100] -> w1090 mode=indexing
            tunnel: [w1099] -> w1093
            tunnel: w1092 -> [w1097]
            tunnel: w1091 -> [w1096]
            n159 = call <vilib>:"Butterworth Filter PtByPt.vi"("initialize"=w1097, "order"=w1096, "filter type"=Filter_Passband_Type."Lowpass", "low cutoff freq: fl"=w1099, "sampling freq: fs"=w1101, "x"=w1102) -> ("Filtered x"=w1100:dbl)  [unwired: 3 in, 1 out]
          }
        }
        frame 77 {
          n160 = for {
            tunnel: w1103 -> [w1116] mode=indexing
            tunnel: w1108 -> [w1113]
            tunnel: w1109 -> [w1115]
            tunnel: [w1114] -> w1104 mode=indexing
            tunnel: [w1113] -> w1107
            tunnel: w1106 -> [w1111]
            tunnel: w1105 -> [w1110]
            n161 = call <vilib>:"Butterworth Filter PtByPt.vi"("initialize"=w1111, "order"=w1110, "filter type"=Filter_Passband_Type."Lowpass", "low cutoff freq: fl"=w1113, "sampling freq: fs"=w1115, "x"=w1116) -> ("Filtered x"=w1114:dbl)  [unwired: 3 in, 1 out]
          }
        }
        frame 78 {
          n162 = for {
            tunnel: w1117 -> [w1130] mode=indexing
            tunnel: w1122 -> [w1127]
            tunnel: w1123 -> [w1129]
            tunnel: [w1128] -> w1118 mode=indexing
            tunnel: [w1127] -> w1121
            tunnel: w1120 -> [w1125]
            tunnel: w1119 -> [w1124]
            n163 = call <vilib>:"Butterworth Filter PtByPt.vi"("initialize"=w1125, "order"=w1124, "filter type"=Filter_Passband_Type."Lowpass", "low cutoff freq: fl"=w1127, "sampling freq: fs"=w1129, "x"=w1130) -> ("Filtered x"=w1128:dbl)  [unwired: 3 in, 1 out]
          }
        }
        frame 79 {
          n164 = for {
            tunnel: w1131 -> [w1144] mode=indexing
            tunnel: w1136 -> [w1141]
            tunnel: w1137 -> [w1143]
            tunnel: [w1142] -> w1132 mode=indexing
            tunnel: [w1141] -> w1135
            tunnel: w1134 -> [w1139]
            tunnel: w1133 -> [w1138]
            n165 = call <vilib>:"Butterworth Filter PtByPt.vi"("initialize"=w1139, "order"=w1138, "filter type"=Filter_Passband_Type."Lowpass", "low cutoff freq: fl"=w1141, "sampling freq: fs"=w1143, "x"=w1144) -> ("Filtered x"=w1142:dbl)  [unwired: 3 in, 1 out]
          }
        }
        frame 80 {
          n166 = for {
            tunnel: w1145 -> [w1158] mode=indexing
            tunnel: w1150 -> [w1155]
            tunnel: w1151 -> [w1157]
            tunnel: [w1156] -> w1146 mode=indexing
            tunnel: [w1155] -> w1149
            tunnel: w1148 -> [w1153]
            tunnel: w1147 -> [w1152]
            n167 = call <vilib>:"Butterworth Filter PtByPt.vi"("initialize"=w1153, "order"=w1152, "filter type"=Filter_Passband_Type."Lowpass", "low cutoff freq: fl"=w1155, "sampling freq: fs"=w1157, "x"=w1158) -> ("Filtered x"=w1156:dbl)  [unwired: 3 in, 1 out]
          }
        }
        frame 81 {
          n168 = for {
            tunnel: w1159 -> [w1172] mode=indexing
            tunnel: w1164 -> [w1169]
            tunnel: w1165 -> [w1171]
            tunnel: [w1170] -> w1160 mode=indexing
            tunnel: [w1169] -> w1163
            tunnel: w1162 -> [w1167]
            tunnel: w1161 -> [w1166]
            n169 = call <vilib>:"Butterworth Filter PtByPt.vi"("initialize"=w1167, "order"=w1166, "filter type"=Filter_Passband_Type."Lowpass", "low cutoff freq: fl"=w1169, "sampling freq: fs"=w1171, "x"=w1172) -> ("Filtered x"=w1170:dbl)  [unwired: 3 in, 1 out]
          }
        }
        frame 82 {
          n170 = for {
            tunnel: w1173 -> [w1186] mode=indexing
            tunnel: w1178 -> [w1183]
            tunnel: w1179 -> [w1185]
            tunnel: [w1184] -> w1174 mode=indexing
            tunnel: [w1183] -> w1177
            tunnel: w1176 -> [w1181]
            tunnel: w1175 -> [w1180]
            n171 = call <vilib>:"Butterworth Filter PtByPt.vi"("initialize"=w1181, "order"=w1180, "filter type"=Filter_Passband_Type."Lowpass", "low cutoff freq: fl"=w1183, "sampling freq: fs"=w1185, "x"=w1186) -> ("Filtered x"=w1184:dbl)  [unwired: 3 in, 1 out]
          }
        }
        frame 83 {
          n172 = for {
            tunnel: w1187 -> [w1200] mode=indexing
            tunnel: w1192 -> [w1197]
            tunnel: w1193 -> [w1199]
            tunnel: [w1198] -> w1188 mode=indexing
            tunnel: [w1197] -> w1191
            tunnel: w1190 -> [w1195]
            tunnel: w1189 -> [w1194]
            n173 = call <vilib>:"Butterworth Filter PtByPt.vi"("initialize"=w1195, "order"=w1194, "filter type"=Filter_Passband_Type."Lowpass", "low cutoff freq: fl"=w1197, "sampling freq: fs"=w1199, "x"=w1200) -> ("Filtered x"=w1198:dbl)  [unwired: 3 in, 1 out]
          }
        }
        frame 84 {
          n174 = for {
            tunnel: w1201 -> [w1214] mode=indexing
            tunnel: w1206 -> [w1211]
            tunnel: w1207 -> [w1213]
            tunnel: [w1212] -> w1202 mode=indexing
            tunnel: [w1211] -> w1205
            tunnel: w1204 -> [w1209]
            tunnel: w1203 -> [w1208]
            n175 = call <vilib>:"Butterworth Filter PtByPt.vi"("initialize"=w1209, "order"=w1208, "filter type"=Filter_Passband_Type."Lowpass", "low cutoff freq: fl"=w1211, "sampling freq: fs"=w1213, "x"=w1214) -> ("Filtered x"=w1212:dbl)  [unwired: 3 in, 1 out]
          }
        }
        frame 85 {
          n176 = for {
            tunnel: w1215 -> [w1228] mode=indexing
            tunnel: w1220 -> [w1225]
            tunnel: w1221 -> [w1227]
            tunnel: [w1226] -> w1216 mode=indexing
            tunnel: [w1225] -> w1219
            tunnel: w1218 -> [w1223]
            tunnel: w1217 -> [w1222]
            n177 = call <vilib>:"Butterworth Filter PtByPt.vi"("initialize"=w1223, "order"=w1222, "filter type"=Filter_Passband_Type."Lowpass", "low cutoff freq: fl"=w1225, "sampling freq: fs"=w1227, "x"=w1228) -> ("Filtered x"=w1226:dbl)  [unwired: 3 in, 1 out]
          }
        }
        frame 86 {
          n178 = for {
            tunnel: w1229 -> [w1242] mode=indexing
            tunnel: w1234 -> [w1239]
            tunnel: w1235 -> [w1241]
            tunnel: [w1240] -> w1230 mode=indexing
            tunnel: [w1239] -> w1233
            tunnel: w1232 -> [w1237]
            tunnel: w1231 -> [w1236]
            n179 = call <vilib>:"Butterworth Filter PtByPt.vi"("initialize"=w1237, "order"=w1236, "filter type"=Filter_Passband_Type."Lowpass", "low cutoff freq: fl"=w1239, "sampling freq: fs"=w1241, "x"=w1242) -> ("Filtered x"=w1240:dbl)  [unwired: 3 in, 1 out]
          }
        }
        frame 87 {
          n180 = for {
            tunnel: w1243 -> [w1256] mode=indexing
            tunnel: w1248 -> [w1253]
            tunnel: w1249 -> [w1255]
            tunnel: [w1254] -> w1244 mode=indexing
            tunnel: [w1253] -> w1247
            tunnel: w1246 -> [w1251]
            tunnel: w1245 -> [w1250]
            n181 = call <vilib>:"Butterworth Filter PtByPt.vi"("initialize"=w1251, "order"=w1250, "filter type"=Filter_Passband_Type."Lowpass", "low cutoff freq: fl"=w1253, "sampling freq: fs"=w1255, "x"=w1256) -> ("Filtered x"=w1254:dbl)  [unwired: 3 in, 1 out]
          }
        }
        frame 88 {
          n182 = for {
            tunnel: w1257 -> [w1270] mode=indexing
            tunnel: w1262 -> [w1267]
            tunnel: w1263 -> [w1269]
            tunnel: [w1268] -> w1258 mode=indexing
            tunnel: [w1267] -> w1261
            tunnel: w1260 -> [w1265]
            tunnel: w1259 -> [w1264]
            n183 = call <vilib>:"Butterworth Filter PtByPt.vi"("initialize"=w1265, "order"=w1264, "filter type"=Filter_Passband_Type."Lowpass", "low cutoff freq: fl"=w1267, "sampling freq: fs"=w1269, "x"=w1270) -> ("Filtered x"=w1268:dbl)  [unwired: 3 in, 1 out]
          }
        }
        frame 89 {
          n184 = for {
            tunnel: w1271 -> [w1284] mode=indexing
            tunnel: w1276 -> [w1281]
            tunnel: w1277 -> [w1283]
            tunnel: [w1282] -> w1272 mode=indexing
            tunnel: [w1281] -> w1275
            tunnel: w1274 -> [w1279]
            tunnel: w1273 -> [w1278]
            n185 = call <vilib>:"Butterworth Filter PtByPt.vi"("initialize"=w1279, "order"=w1278, "filter type"=Filter_Passband_Type."Lowpass", "low cutoff freq: fl"=w1281, "sampling freq: fs"=w1283, "x"=w1284) -> ("Filtered x"=w1282:dbl)  [unwired: 3 in, 1 out]
          }
        }
        frame 90 {
          n186 = for {
            tunnel: w1285 -> [w1298] mode=indexing
            tunnel: w1290 -> [w1295]
            tunnel: w1291 -> [w1297]
            tunnel: [w1296] -> w1286 mode=indexing
            tunnel: [w1295] -> w1289
            tunnel: w1288 -> [w1293]
            tunnel: w1287 -> [w1292]
            n187 = call <vilib>:"Butterworth Filter PtByPt.vi"("initialize"=w1293, "order"=w1292, "filter type"=Filter_Passband_Type."Lowpass", "low cutoff freq: fl"=w1295, "sampling freq: fs"=w1297, "x"=w1298) -> ("Filtered x"=w1296:dbl)  [unwired: 3 in, 1 out]
          }
        }
        frame 91 {
          n188 = for {
            tunnel: w1299 -> [w1312] mode=indexing
            tunnel: w1304 -> [w1309]
            tunnel: w1305 -> [w1311]
            tunnel: [w1310] -> w1300 mode=indexing
            tunnel: [w1309] -> w1303
            tunnel: w1302 -> [w1307]
            tunnel: w1301 -> [w1306]
            n189 = call <vilib>:"Butterworth Filter PtByPt.vi"("initialize"=w1307, "order"=w1306, "filter type"=Filter_Passband_Type."Lowpass", "low cutoff freq: fl"=w1309, "sampling freq: fs"=w1311, "x"=w1312) -> ("Filtered x"=w1310:dbl)  [unwired: 3 in, 1 out]
          }
        }
        frame 92 {
          n190 = for {
            tunnel: w1313 -> [w1326] mode=indexing
            tunnel: w1318 -> [w1323]
            tunnel: w1319 -> [w1325]
            tunnel: [w1324] -> w1314 mode=indexing
            tunnel: [w1323] -> w1317
            tunnel: w1316 -> [w1321]
            tunnel: w1315 -> [w1320]
            n191 = call <vilib>:"Butterworth Filter PtByPt.vi"("initialize"=w1321, "order"=w1320, "filter type"=Filter_Passband_Type."Lowpass", "low cutoff freq: fl"=w1323, "sampling freq: fs"=w1325, "x"=w1326) -> ("Filtered x"=w1324:dbl)  [unwired: 3 in, 1 out]
          }
        }
        frame 93 {
          n192 = for {
            tunnel: w1327 -> [w1340] mode=indexing
            tunnel: w1332 -> [w1337]
            tunnel: w1333 -> [w1339]
            tunnel: [w1338] -> w1328 mode=indexing
            tunnel: [w1337] -> w1331
            tunnel: w1330 -> [w1335]
            tunnel: w1329 -> [w1334]
            n193 = call <vilib>:"Butterworth Filter PtByPt.vi"("initialize"=w1335, "order"=w1334, "filter type"=Filter_Passband_Type."Lowpass", "low cutoff freq: fl"=w1337, "sampling freq: fs"=w1339, "x"=w1340) -> ("Filtered x"=w1338:dbl)  [unwired: 3 in, 1 out]
          }
        }
        frame 94 {
          n194 = for {
            tunnel: w1341 -> [w1354] mode=indexing
            tunnel: w1346 -> [w1351]
            tunnel: w1347 -> [w1353]
            tunnel: [w1352] -> w1342 mode=indexing
            tunnel: [w1351] -> w1345
            tunnel: w1344 -> [w1349]
            tunnel: w1343 -> [w1348]
            n195 = call <vilib>:"Butterworth Filter PtByPt.vi"("initialize"=w1349, "order"=w1348, "filter type"=Filter_Passband_Type."Lowpass", "low cutoff freq: fl"=w1351, "sampling freq: fs"=w1353, "x"=w1354) -> ("Filtered x"=w1352:dbl)  [unwired: 3 in, 1 out]
          }
        }
        frame 95 {
          n196 = for {
            tunnel: w1355 -> [w1368] mode=indexing
            tunnel: w1360 -> [w1365]
            tunnel: w1361 -> [w1367]
            tunnel: [w1366] -> w1356 mode=indexing
            tunnel: [w1365] -> w1359
            tunnel: w1358 -> [w1363]
            tunnel: w1357 -> [w1362]
            n197 = call <vilib>:"Butterworth Filter PtByPt.vi"("initialize"=w1363, "order"=w1362, "filter type"=Filter_Passband_Type."Lowpass", "low cutoff freq: fl"=w1365, "sampling freq: fs"=w1367, "x"=w1368) -> ("Filtered x"=w1366:dbl)  [unwired: 3 in, 1 out]
          }
        }
        frame 96 {
          n198 = for {
            tunnel: w1369 -> [w1382] mode=indexing
            tunnel: w1374 -> [w1379]
            tunnel: w1375 -> [w1381]
            tunnel: [w1380] -> w1370 mode=indexing
            tunnel: [w1379] -> w1373
            tunnel: w1372 -> [w1377]
            tunnel: w1371 -> [w1376]
            n199 = call <vilib>:"Butterworth Filter PtByPt.vi"("initialize"=w1377, "order"=w1376, "filter type"=Filter_Passband_Type."Lowpass", "low cutoff freq: fl"=w1379, "sampling freq: fs"=w1381, "x"=w1382) -> ("Filtered x"=w1380:dbl)  [unwired: 3 in, 1 out]
          }
        }
        frame 97 {
          n200 = for {
            tunnel: w1383 -> [w1396] mode=indexing
            tunnel: w1388 -> [w1393]
            tunnel: w1389 -> [w1395]
            tunnel: [w1394] -> w1384 mode=indexing
            tunnel: [w1393] -> w1387
            tunnel: w1386 -> [w1391]
            tunnel: w1385 -> [w1390]
            n201 = call <vilib>:"Butterworth Filter PtByPt.vi"("initialize"=w1391, "order"=w1390, "filter type"=Filter_Passband_Type."Lowpass", "low cutoff freq: fl"=w1393, "sampling freq: fs"=w1395, "x"=w1396) -> ("Filtered x"=w1394:dbl)  [unwired: 3 in, 1 out]
          }
        }
        frame 98 {
          n202 = for {
            tunnel: w1397 -> [w1410] mode=indexing
            tunnel: w1402 -> [w1407]
            tunnel: w1403 -> [w1409]
            tunnel: [w1408] -> w1398 mode=indexing
            tunnel: [w1407] -> w1401
            tunnel: w1400 -> [w1405]
            tunnel: w1399 -> [w1404]
            n203 = call <vilib>:"Butterworth Filter PtByPt.vi"("initialize"=w1405, "order"=w1404, "filter type"=Filter_Passband_Type."Lowpass", "low cutoff freq: fl"=w1407, "sampling freq: fs"=w1409, "x"=w1410) -> ("Filtered x"=w1408:dbl)  [unwired: 3 in, 1 out]
          }
        }
        frame 99 {
          n204 = for {
            tunnel: w1411 -> [w1424] mode=indexing
            tunnel: w1416 -> [w1421]
            tunnel: w1417 -> [w1423]
            tunnel: [w1422] -> w1412 mode=indexing
            tunnel: [w1421] -> w1415
            tunnel: w1414 -> [w1419]
            tunnel: w1413 -> [w1418]
            n205 = call <vilib>:"Butterworth Filter PtByPt.vi"("initialize"=w1419, "order"=w1418, "filter type"=Filter_Passband_Type."Lowpass", "low cutoff freq: fl"=w1421, "sampling freq: fs"=w1423, "x"=w1424) -> ("Filtered x"=w1422:dbl)  [unwired: 3 in, 1 out]
          }
        }
        frame 100 {
          n206 = for {
            tunnel: w1425 -> [w1438] mode=indexing
            tunnel: w1430 -> [w1435]
            tunnel: w1431 -> [w1437]
            tunnel: [w1436] -> w1426 mode=indexing
            tunnel: [w1435] -> w1429
            tunnel: w1428 -> [w1433]
            tunnel: w1427 -> [w1432]
            n207 = call <vilib>:"Butterworth Filter PtByPt.vi"("initialize"=w1433, "order"=w1432, "filter type"=Filter_Passband_Type."Lowpass", "low cutoff freq: fl"=w1435, "sampling freq: fs"=w1437, "x"=w1438) -> ("Filtered x"=w1436:dbl)  [unwired: 3 in, 1 out]
          }
        }
        frame 101 {
          n208 = for {
            tunnel: w1439 -> [w1452] mode=indexing
            tunnel: w1444 -> [w1449]
            tunnel: w1445 -> [w1451]
            tunnel: [w1450] -> w1440 mode=indexing
            tunnel: [w1449] -> w1443
            tunnel: w1442 -> [w1447]
            tunnel: w1441 -> [w1446]
            n209 = call <vilib>:"Butterworth Filter PtByPt.vi"("initialize"=w1447, "order"=w1446, "filter type"=Filter_Passband_Type."Lowpass", "low cutoff freq: fl"=w1449, "sampling freq: fs"=w1451, "x"=w1452) -> ("Filtered x"=w1450:dbl)  [unwired: 3 in, 1 out]
          }
        }
        frame 102 {
          n210 = for {
            tunnel: w1453 -> [w1466] mode=indexing
            tunnel: w1458 -> [w1463]
            tunnel: w1459 -> [w1465]
            tunnel: [w1464] -> w1454 mode=indexing
            tunnel: [w1463] -> w1457
            tunnel: w1456 -> [w1461]
            tunnel: w1455 -> [w1460]
            n211 = call <vilib>:"Butterworth Filter PtByPt.vi"("initialize"=w1461, "order"=w1460, "filter type"=Filter_Passband_Type."Lowpass", "low cutoff freq: fl"=w1463, "sampling freq: fs"=w1465, "x"=w1466) -> ("Filtered x"=w1464:dbl)  [unwired: 3 in, 1 out]
          }
        }
        frame 103 {
          n212 = for {
            tunnel: w1467 -> [w1480] mode=indexing
            tunnel: w1472 -> [w1477]
            tunnel: w1473 -> [w1479]
            tunnel: [w1478] -> w1468 mode=indexing
            tunnel: [w1477] -> w1471
            tunnel: w1470 -> [w1475]
            tunnel: w1469 -> [w1474]
            n213 = call <vilib>:"Butterworth Filter PtByPt.vi"("initialize"=w1475, "order"=w1474, "filter type"=Filter_Passband_Type."Lowpass", "low cutoff freq: fl"=w1477, "sampling freq: fs"=w1479, "x"=w1480) -> ("Filtered x"=w1478:dbl)  [unwired: 3 in, 1 out]
          }
        }
        frame 104 {
          n214 = for {
            tunnel: w1481 -> [w1494] mode=indexing
            tunnel: w1486 -> [w1491]
            tunnel: w1487 -> [w1493]
            tunnel: [w1492] -> w1482 mode=indexing
            tunnel: [w1491] -> w1485
            tunnel: w1484 -> [w1489]
            tunnel: w1483 -> [w1488]
            n215 = call <vilib>:"Butterworth Filter PtByPt.vi"("initialize"=w1489, "order"=w1488, "filter type"=Filter_Passband_Type."Lowpass", "low cutoff freq: fl"=w1491, "sampling freq: fs"=w1493, "x"=w1494) -> ("Filtered x"=w1492:dbl)  [unwired: 3 in, 1 out]
          }
        }
        frame 105 {
          n216 = for {
            tunnel: w1495 -> [w1508] mode=indexing
            tunnel: w1500 -> [w1505]
            tunnel: w1501 -> [w1507]
            tunnel: [w1506] -> w1496 mode=indexing
            tunnel: [w1505] -> w1499
            tunnel: w1498 -> [w1503]
            tunnel: w1497 -> [w1502]
            n217 = call <vilib>:"Butterworth Filter PtByPt.vi"("initialize"=w1503, "order"=w1502, "filter type"=Filter_Passband_Type."Lowpass", "low cutoff freq: fl"=w1505, "sampling freq: fs"=w1507, "x"=w1508) -> ("Filtered x"=w1506:dbl)  [unwired: 3 in, 1 out]
          }
        }
        frame 106 {
          n218 = for {
            tunnel: w1509 -> [w1522] mode=indexing
            tunnel: w1514 -> [w1519]
            tunnel: w1515 -> [w1521]
            tunnel: [w1520] -> w1510 mode=indexing
            tunnel: [w1519] -> w1513
            tunnel: w1512 -> [w1517]
            tunnel: w1511 -> [w1516]
            n219 = call <vilib>:"Butterworth Filter PtByPt.vi"("initialize"=w1517, "order"=w1516, "filter type"=Filter_Passband_Type."Lowpass", "low cutoff freq: fl"=w1519, "sampling freq: fs"=w1521, "x"=w1522) -> ("Filtered x"=w1520:dbl)  [unwired: 3 in, 1 out]
          }
        }
        frame 107 {
          n220 = for {
            tunnel: w1523 -> [w1536] mode=indexing
            tunnel: w1528 -> [w1533]
            tunnel: w1529 -> [w1535]
            tunnel: [w1534] -> w1524 mode=indexing
            tunnel: [w1533] -> w1527
            tunnel: w1526 -> [w1531]
            tunnel: w1525 -> [w1530]
            n221 = call <vilib>:"Butterworth Filter PtByPt.vi"("initialize"=w1531, "order"=w1530, "filter type"=Filter_Passband_Type."Lowpass", "low cutoff freq: fl"=w1533, "sampling freq: fs"=w1535, "x"=w1536) -> ("Filtered x"=w1534:dbl)  [unwired: 3 in, 1 out]
          }
        }
        frame 108 {
          n222 = for {
            tunnel: w1537 -> [w1550] mode=indexing
            tunnel: w1542 -> [w1547]
            tunnel: w1543 -> [w1549]
            tunnel: [w1548] -> w1538 mode=indexing
            tunnel: [w1547] -> w1541
            tunnel: w1540 -> [w1545]
            tunnel: w1539 -> [w1544]
            n223 = call <vilib>:"Butterworth Filter PtByPt.vi"("initialize"=w1545, "order"=w1544, "filter type"=Filter_Passband_Type."Lowpass", "low cutoff freq: fl"=w1547, "sampling freq: fs"=w1549, "x"=w1550) -> ("Filtered x"=w1548:dbl)  [unwired: 3 in, 1 out]
          }
        }
        frame 109 {
          n224 = for {
            tunnel: w1551 -> [w1564] mode=indexing
            tunnel: w1556 -> [w1561]
            tunnel: w1557 -> [w1563]
            tunnel: [w1562] -> w1552 mode=indexing
            tunnel: [w1561] -> w1555
            tunnel: w1554 -> [w1559]
            tunnel: w1553 -> [w1558]
            n225 = call <vilib>:"Butterworth Filter PtByPt.vi"("initialize"=w1559, "order"=w1558, "filter type"=Filter_Passband_Type."Lowpass", "low cutoff freq: fl"=w1561, "sampling freq: fs"=w1563, "x"=w1564) -> ("Filtered x"=w1562:dbl)  [unwired: 3 in, 1 out]
          }
        }
        frame 110 {
          n226 = for {
            tunnel: w1565 -> [w1578] mode=indexing
            tunnel: w1570 -> [w1575]
            tunnel: w1571 -> [w1577]
            tunnel: [w1576] -> w1566 mode=indexing
            tunnel: [w1575] -> w1569
            tunnel: w1568 -> [w1573]
            tunnel: w1567 -> [w1572]
            n227 = call <vilib>:"Butterworth Filter PtByPt.vi"("initialize"=w1573, "order"=w1572, "filter type"=Filter_Passband_Type."Lowpass", "low cutoff freq: fl"=w1575, "sampling freq: fs"=w1577, "x"=w1578) -> ("Filtered x"=w1576:dbl)  [unwired: 3 in, 1 out]
          }
        }
        frame 111 {
          n228 = for {
            tunnel: w1579 -> [w1592] mode=indexing
            tunnel: w1584 -> [w1589]
            tunnel: w1585 -> [w1591]
            tunnel: [w1590] -> w1580 mode=indexing
            tunnel: [w1589] -> w1583
            tunnel: w1582 -> [w1587]
            tunnel: w1581 -> [w1586]
            n229 = call <vilib>:"Butterworth Filter PtByPt.vi"("initialize"=w1587, "order"=w1586, "filter type"=Filter_Passband_Type."Lowpass", "low cutoff freq: fl"=w1589, "sampling freq: fs"=w1591, "x"=w1592) -> ("Filtered x"=w1590:dbl)  [unwired: 3 in, 1 out]
          }
        }
        frame 112 {
          n230 = for {
            tunnel: w1593 -> [w1606] mode=indexing
            tunnel: w1598 -> [w1603]
            tunnel: w1599 -> [w1605]
            tunnel: [w1604] -> w1594 mode=indexing
            tunnel: [w1603] -> w1597
            tunnel: w1596 -> [w1601]
            tunnel: w1595 -> [w1600]
            n231 = call <vilib>:"Butterworth Filter PtByPt.vi"("initialize"=w1601, "order"=w1600, "filter type"=Filter_Passband_Type."Lowpass", "low cutoff freq: fl"=w1603, "sampling freq: fs"=w1605, "x"=w1606) -> ("Filtered x"=w1604:dbl)  [unwired: 3 in, 1 out]
          }
        }
        frame 113 {
          n232 = for {
            tunnel: w1607 -> [w1620] mode=indexing
            tunnel: w1612 -> [w1617]
            tunnel: w1613 -> [w1619]
            tunnel: [w1618] -> w1608 mode=indexing
            tunnel: [w1617] -> w1611
            tunnel: w1610 -> [w1615]
            tunnel: w1609 -> [w1614]
            n233 = call <vilib>:"Butterworth Filter PtByPt.vi"("initialize"=w1615, "order"=w1614, "filter type"=Filter_Passband_Type."Lowpass", "low cutoff freq: fl"=w1617, "sampling freq: fs"=w1619, "x"=w1620) -> ("Filtered x"=w1618:dbl)  [unwired: 3 in, 1 out]
          }
        }
        frame 114 {
          n234 = for {
            tunnel: w1621 -> [w1634] mode=indexing
            tunnel: w1626 -> [w1631]
            tunnel: w1627 -> [w1633]
            tunnel: [w1632] -> w1622 mode=indexing
            tunnel: [w1631] -> w1625
            tunnel: w1624 -> [w1629]
            tunnel: w1623 -> [w1628]
            n235 = call <vilib>:"Butterworth Filter PtByPt.vi"("initialize"=w1629, "order"=w1628, "filter type"=Filter_Passband_Type."Lowpass", "low cutoff freq: fl"=w1631, "sampling freq: fs"=w1633, "x"=w1634) -> ("Filtered x"=w1632:dbl)  [unwired: 3 in, 1 out]
          }
        }
        frame 115 {
          n236 = for {
            tunnel: w1635 -> [w1648] mode=indexing
            tunnel: w1640 -> [w1645]
            tunnel: w1641 -> [w1647]
            tunnel: [w1646] -> w1636 mode=indexing
            tunnel: [w1645] -> w1639
            tunnel: w1638 -> [w1643]
            tunnel: w1637 -> [w1642]
            n237 = call <vilib>:"Butterworth Filter PtByPt.vi"("initialize"=w1643, "order"=w1642, "filter type"=Filter_Passband_Type."Lowpass", "low cutoff freq: fl"=w1645, "sampling freq: fs"=w1647, "x"=w1648) -> ("Filtered x"=w1646:dbl)  [unwired: 3 in, 1 out]
          }
        }
        frame 116 {
          n238 = for {
            tunnel: w1649 -> [w1662] mode=indexing
            tunnel: w1654 -> [w1659]
            tunnel: w1655 -> [w1661]
            tunnel: [w1660] -> w1650 mode=indexing
            tunnel: [w1659] -> w1653
            tunnel: w1652 -> [w1657]
            tunnel: w1651 -> [w1656]
            n239 = call <vilib>:"Butterworth Filter PtByPt.vi"("initialize"=w1657, "order"=w1656, "filter type"=Filter_Passband_Type."Lowpass", "low cutoff freq: fl"=w1659, "sampling freq: fs"=w1661, "x"=w1662) -> ("Filtered x"=w1660:dbl)  [unwired: 3 in, 1 out]
          }
        }
        frame 117 {
          n240 = for {
            tunnel: w1663 -> [w1676] mode=indexing
            tunnel: w1668 -> [w1673]
            tunnel: w1669 -> [w1675]
            tunnel: [w1674] -> w1664 mode=indexing
            tunnel: [w1673] -> w1667
            tunnel: w1666 -> [w1671]
            tunnel: w1665 -> [w1670]
            n241 = call <vilib>:"Butterworth Filter PtByPt.vi"("initialize"=w1671, "order"=w1670, "filter type"=Filter_Passband_Type."Lowpass", "low cutoff freq: fl"=w1673, "sampling freq: fs"=w1675, "x"=w1676) -> ("Filtered x"=w1674:dbl)  [unwired: 3 in, 1 out]
          }
        }
        frame 118 {
          n242 = for {
            tunnel: w1677 -> [w1690] mode=indexing
            tunnel: w1682 -> [w1687]
            tunnel: w1683 -> [w1689]
            tunnel: [w1688] -> w1678 mode=indexing
            tunnel: [w1687] -> w1681
            tunnel: w1680 -> [w1685]
            tunnel: w1679 -> [w1684]
            n243 = call <vilib>:"Butterworth Filter PtByPt.vi"("initialize"=w1685, "order"=w1684, "filter type"=Filter_Passband_Type."Lowpass", "low cutoff freq: fl"=w1687, "sampling freq: fs"=w1689, "x"=w1690) -> ("Filtered x"=w1688:dbl)  [unwired: 3 in, 1 out]
          }
        }
        frame 119 {
          n244 = for {
            tunnel: w1691 -> [w1704] mode=indexing
            tunnel: w1696 -> [w1701]
            tunnel: w1697 -> [w1703]
            tunnel: [w1702] -> w1692 mode=indexing
            tunnel: [w1701] -> w1695
            tunnel: w1694 -> [w1699]
            tunnel: w1693 -> [w1698]
            n245 = call <vilib>:"Butterworth Filter PtByPt.vi"("initialize"=w1699, "order"=w1698, "filter type"=Filter_Passband_Type."Lowpass", "low cutoff freq: fl"=w1701, "sampling freq: fs"=w1703, "x"=w1704) -> ("Filtered x"=w1702:dbl)  [unwired: 3 in, 1 out]
          }
        }
        frame 120 {
          n246 = for {
            tunnel: w1705 -> [w1718] mode=indexing
            tunnel: w1710 -> [w1715]
            tunnel: w1711 -> [w1717]
            tunnel: [w1716] -> w1706 mode=indexing
            tunnel: [w1715] -> w1709
            tunnel: w1708 -> [w1713]
            tunnel: w1707 -> [w1712]
            n247 = call <vilib>:"Butterworth Filter PtByPt.vi"("initialize"=w1713, "order"=w1712, "filter type"=Filter_Passband_Type."Lowpass", "low cutoff freq: fl"=w1715, "sampling freq: fs"=w1717, "x"=w1718) -> ("Filtered x"=w1716:dbl)  [unwired: 3 in, 1 out]
          }
        }
        frame 121 {
          n248 = for {
            tunnel: w1719 -> [w1732] mode=indexing
            tunnel: w1724 -> [w1729]
            tunnel: w1725 -> [w1731]
            tunnel: [w1730] -> w1720 mode=indexing
            tunnel: [w1729] -> w1723
            tunnel: w1722 -> [w1727]
            tunnel: w1721 -> [w1726]
            n249 = call <vilib>:"Butterworth Filter PtByPt.vi"("initialize"=w1727, "order"=w1726, "filter type"=Filter_Passband_Type."Lowpass", "low cutoff freq: fl"=w1729, "sampling freq: fs"=w1731, "x"=w1732) -> ("Filtered x"=w1730:dbl)  [unwired: 3 in, 1 out]
          }
        }
        frame 122 {
          n250 = for {
            tunnel: w1733 -> [w1746] mode=indexing
            tunnel: w1738 -> [w1743]
            tunnel: w1739 -> [w1745]
            tunnel: [w1744] -> w1734 mode=indexing
            tunnel: [w1743] -> w1737
            tunnel: w1736 -> [w1741]
            tunnel: w1735 -> [w1740]
            n251 = call <vilib>:"Butterworth Filter PtByPt.vi"("initialize"=w1741, "order"=w1740, "filter type"=Filter_Passband_Type."Lowpass", "low cutoff freq: fl"=w1743, "sampling freq: fs"=w1745, "x"=w1746) -> ("Filtered x"=w1744:dbl)  [unwired: 3 in, 1 out]
          }
        }
        frame 123 {
          n252 = for {
            tunnel: w1747 -> [w1760] mode=indexing
            tunnel: w1752 -> [w1757]
            tunnel: w1753 -> [w1759]
            tunnel: [w1758] -> w1748 mode=indexing
            tunnel: [w1757] -> w1751
            tunnel: w1750 -> [w1755]
            tunnel: w1749 -> [w1754]
            n253 = call <vilib>:"Butterworth Filter PtByPt.vi"("initialize"=w1755, "order"=w1754, "filter type"=Filter_Passband_Type."Lowpass", "low cutoff freq: fl"=w1757, "sampling freq: fs"=w1759, "x"=w1760) -> ("Filtered x"=w1758:dbl)  [unwired: 3 in, 1 out]
          }
        }
      }
      n254 = Bundle By Name(cluster=w22, "Y"=w17) -> (w23:waveform(dbl))
    }
  }
  "Array out" <- w4
